vi "Protype 1.1.vi"() -> ()   [LabVIEW 2020]
uses:
  <vilib>/Utility/error.llb/DialogType.ctl
panel:
  out "MQ4 - 2":cluster{"X":dbl[], "Y":dbl[]}[](graph)
  out "MQ3 - 2":cluster{"X":dbl[], "Y":dbl[]}[](graph)
  out "Temperatur - 2":cluster{"X":dbl[], "Y":dbl[]}[](graph)
  out "Luftfeuchtigkeit - 2":cluster{"X":dbl[], "Y":dbl[]}[](graph)
  out "RAW Ethanol - 2":cluster{"X":dbl[], "Y":dbl[]}[](graph)
  out "RAW H2 - 2":cluster{"X":dbl[], "Y":dbl[]}[](graph)
  out "TVOC - 2":cluster{"X":dbl[], "Y":dbl[]}[](graph)
  out "x-y 6":dbl
  out "eCO2 - 2":cluster{"X":dbl[], "Y":dbl[]}[](graph)
  out "MH-Z19B - 2":cluster{"X":dbl[], "Y":dbl[]}[](graph)
  out "x-y 5":dbl
  out "Vernier CO2  - 2":cluster{"X":dbl[], "Y":dbl[]}[](graph) caption="XY-Graph"
  out "x-y 4":dbl
  out "Vernier Spirometer - 2":cluster{"X":dbl[], "Y":dbl[]}[](graph)
  out "x-y 3":dbl
  out "Vernier O2 - 2":cluster{"X":dbl[], "Y":dbl[]}[](graph)
  out "x-y 2":dbl
  out "Waage 2":cluster{"X":dbl[], "Y":dbl[]}[](graph) caption="XY-Graph"
  in  "Switch":bool
  in  "Graph Range":dbl=30.0
  out "x-y":dbl
  out "Luftfeuchtigkeit":dbl
  out "Temperatur":dbl
  out "Temperatur":cluster{"Y":dbl[], "Y":dbl[]}[](graph)
  out "MQ4":dbl
  out "MQ3":dbl
  out "RAW Ethanol":dbl
  out "RAW H2":dbl
  out "TVOC":dbl
  out "eCO2":dbl
  out "MHZ19b":dbl
  out "Vernier CO2":dbl
  out "Vernier Spirometer":dbl
  out "Vernier O2":dbl
  out "Waage":dbl
  in  "Filename":path=path "Komplett.xlsx" caption="Dateiname"
  in  "Record interval [ms]":u32=10000
  out "error out":errorcluster caption="Fehler (Ausgang)"
  in  "Record ?":bool=TRUE
  out "General Settings:Maximum Queue Length":u32
  out "HEMTLL - Arraygröße":i32
  out "Current Value HEMTLL":dbl[](array[numeric])
  out "Data Storage Vector - HEMTLL":dbl[][](array[numeric])
  in  "Reset MQ4":bool
  in  "Reset MQ3":bool
  in  "Reset Luftfeuchtigkeit":bool
  in  "Reset RAW Ethanol":bool
  in  "Reset RAW H2":bool
  in  "reset TVOC":bool
  in  "reset eCO2":bool
  out "Elapsed Time [s]":dbl
  out "Fehlermeldungen 8":string=" ANWEISUNGEN:\r\rAllgemeine Nutzung:  Bei der Benutzung von SubVIs, die mit den Anschlüssen \"Fehler(Eingang)\" und \"Fehler(Ausgang)\" arbeiten, platzieren Sie diesen Handler dort, wo Sie den Benutzer auf aufgetretene Fehler hinweisen möchten. In der Regel wird er am Ende eines Datenpfads als letzte Aktion des Programms aufgerufen.  Wenn der Fehlerstatus einen Fehler angibt, erzeugt der Handler eine Nachricht, die den Fehler und dessen Ursprung beschreibt.  Ist Dialogtyp = 1 (Standardeinstellung), wird die Fehlermeldung angezeigt und der Benutzer kann diese bestätigen.  Ist Dialogtyp = 2, kann der Benutzer die Meldung bestätigen oder die Programmausführung abbrechen. Der Abbruch eines Programms mit aktiver I/O wird jedoch nicht empfohlen.  Ist der Dialogtyp = 0, wird keine Meldung angezeigt; dieser Modus wird verwendet, um Fehler programmatisch zu behandeln. Aus diesem Grunde sind auch die Fehlerausgangs-Cluster mit individuellen Anschlüssen verbunden.  \r\rAndere Nutzungsmöglichkeit:\n\r\nLokales Testen.  Um einen Fehlercode eines SubVIs oder einer Funktion zu testen, die nicht mit den Fehleranschlüssen arbeitet, können der Fehlercode und ein String für \"Quelle\" mit den lokalen Eingängen \"Fehlercode\" und \"Quelle\" verbunden werden.  Wenn der Fehlerstatus keinen Fehler anzeigt und der Fehlercode ungleich 0 ist, werden der lokale Code und String \"Quelle\" ersetzt und \"Fehler?\" lautet TRUE (FEHLER)." caption="HEMTTL - Error"
  out "Gelöschte Elemente\nHEMTTL":dbl[][](array[numeric])
  out "MQ4":cluster{"Y":dbl[], "Y":dbl[]}[](graph)
  out "MQ3":cluster{"Y":dbl[], "Y":dbl[]}[](graph)
  out "Luftfeuchtigkeit":cluster{"Y":dbl[], "Y":dbl[]}[](graph)
  out "RAW Ethanol":cluster{"Y":dbl[], "Y":dbl[]}[](graph)
  out "RAW H2":cluster{"Y":dbl[], "Y":dbl[]}[](graph)
  out "TVOC":cluster{"Y":dbl[], "Y":dbl[]}[](graph)
  out "eCO2":cluster{"Y":dbl[], "Y":dbl[]}[](graph)
  in  "HEMTTL":refnum<visa-resource-name>="COM23"
  out "Vernier O2":cluster{"X":dbl[], "Y":dbl[]}[](graph) caption="XY-Graph"
  out "Gelöschte Elemente \nVernier O2":dbl[][](array[numeric])
  out "Vernier O2 - Data Storage Vector":dbl[][](array[numeric])
  out "Current Value - Vernier O2":dbl[](array[numeric])
  out "Vernier O2":i32
  in  "Reset Vernier O2":bool caption="Zurücksetzen"
  out "Fehlermeldungen 7":string=" ANWEISUNGEN:\r\rAllgemeine Nutzung:  Bei der Benutzung von SubVIs, die mit den Anschlüssen \"Fehler(Eingang)\" und \"Fehler(Ausgang)\" arbeiten, platzieren Sie diesen Handler dort, wo Sie den Benutzer auf aufgetretene Fehler hinweisen möchten. In der Regel wird er am Ende eines Datenpfads als letzte Aktion des Programms aufgerufen.  Wenn der Fehlerstatus einen Fehler angibt, erzeugt der Handler eine Nachricht, die den Fehler und dessen Ursprung beschreibt.  Ist Dialogtyp = 1 (Standardeinstellung), wird die Fehlermeldung angezeigt und der Benutzer kann diese bestätigen.  Ist Dialogtyp = 2, kann der Benutzer die Meldung bestätigen oder die Programmausführung abbrechen. Der Abbruch eines Programms mit aktiver I/O wird jedoch nicht empfohlen.  Ist der Dialogtyp = 0, wird keine Meldung angezeigt; dieser Modus wird verwendet, um Fehler programmatisch zu behandeln. Aus diesem Grunde sind auch die Fehlerausgangs-Cluster mit individuellen Anschlüssen verbunden.  \r\rAndere Nutzungsmöglichkeit:\n\r\nLokales Testen.  Um einen Fehlercode eines SubVIs oder einer Funktion zu testen, die nicht mit den Fehleranschlüssen arbeitet, können der Fehlercode und ein String für \"Quelle\" mit den lokalen Eingängen \"Fehlercode\" und \"Quelle\" verbunden werden.  Wenn der Fehlerstatus keinen Fehler anzeigt und der Fehlercode ungleich 0 ist, werden der lokale Code und String \"Quelle\" ersetzt und \"Fehler?\" lautet TRUE (FEHLER)."
  out "Vernier Spirometer":cluster{"X":dbl[], "Y":dbl[]}[](graph) caption="XY-Graph"
  out "Gelöschte Elemente \nVernier Spirometer":dbl[][](array[numeric])
  out "Data Storage vector - \nVernier Spirometer":dbl[][](array[numeric])
  out "Current Value - \nVernier Spirometer":dbl[](array[numeric])
  out "Vernier Spirometer-\n Array Größe":i32
  in  "Reset Spirometer":bool caption="Zurücksetzen"
  out "Fehlermeldungen 6":string=" ANWEISUNGEN:\r\rAllgemeine Nutzung:  Bei der Benutzung von SubVIs, die mit den Anschlüssen \"Fehler(Eingang)\" und \"Fehler(Ausgang)\" arbeiten, platzieren Sie diesen Handler dort, wo Sie den Benutzer auf aufgetretene Fehler hinweisen möchten. In der Regel wird er am Ende eines Datenpfads als letzte Aktion des Programms aufgerufen.  Wenn der Fehlerstatus einen Fehler angibt, erzeugt der Handler eine Nachricht, die den Fehler und dessen Ursprung beschreibt.  Ist Dialogtyp = 1 (Standardeinstellung), wird die Fehlermeldung angezeigt und der Benutzer kann diese bestätigen.  Ist Dialogtyp = 2, kann der Benutzer die Meldung bestätigen oder die Programmausführung abbrechen. Der Abbruch eines Programms mit aktiver I/O wird jedoch nicht empfohlen.  Ist der Dialogtyp = 0, wird keine Meldung angezeigt; dieser Modus wird verwendet, um Fehler programmatisch zu behandeln. Aus diesem Grunde sind auch die Fehlerausgangs-Cluster mit individuellen Anschlüssen verbunden.  \r\rAndere Nutzungsmöglichkeit:\n\r\nLokales Testen.  Um einen Fehlercode eines SubVIs oder einer Funktion zu testen, die nicht mit den Fehleranschlüssen arbeitet, können der Fehlercode und ein String für \"Quelle\" mit den lokalen Eingängen \"Fehlercode\" und \"Quelle\" verbunden werden.  Wenn der Fehlerstatus keinen Fehler anzeigt und der Fehlercode ungleich 0 ist, werden der lokale Code und String \"Quelle\" ersetzt und \"Fehler?\" lautet TRUE (FEHLER)."
  out "MH-Z19B":cluster{"X":dbl[], "Y":dbl[]}[](graph) caption="XY-Graph"
  out "Gelöschte Elemente \nMHZ19b":dbl[][](array[numeric])
  out "MHZ19b":dbl[][](array[numeric])
  out "Current Value - MHZ19b":dbl[](array[numeric])
  out "MHZ19b - Arraygröße":i32
  in  "Reset MHZ19b":bool caption="Zurücksetzen"
  out "Fehlermeldungen 5":string=" ANWEISUNGEN:\r\rAllgemeine Nutzung:  Bei der Benutzung von SubVIs, die mit den Anschlüssen \"Fehler(Eingang)\" und \"Fehler(Ausgang)\" arbeiten, platzieren Sie diesen Handler dort, wo Sie den Benutzer auf aufgetretene Fehler hinweisen möchten. In der Regel wird er am Ende eines Datenpfads als letzte Aktion des Programms aufgerufen.  Wenn der Fehlerstatus einen Fehler angibt, erzeugt der Handler eine Nachricht, die den Fehler und dessen Ursprung beschreibt.  Ist Dialogtyp = 1 (Standardeinstellung), wird die Fehlermeldung angezeigt und der Benutzer kann diese bestätigen.  Ist Dialogtyp = 2, kann der Benutzer die Meldung bestätigen oder die Programmausführung abbrechen. Der Abbruch eines Programms mit aktiver I/O wird jedoch nicht empfohlen.  Ist der Dialogtyp = 0, wird keine Meldung angezeigt; dieser Modus wird verwendet, um Fehler programmatisch zu behandeln. Aus diesem Grunde sind auch die Fehlerausgangs-Cluster mit individuellen Anschlüssen verbunden.  \r\rAndere Nutzungsmöglichkeit:\n\r\nLokales Testen.  Um einen Fehlercode eines SubVIs oder einer Funktion zu testen, die nicht mit den Fehleranschlüssen arbeitet, können der Fehlercode und ein String für \"Quelle\" mit den lokalen Eingängen \"Fehlercode\" und \"Quelle\" verbunden werden.  Wenn der Fehlerstatus keinen Fehler anzeigt und der Fehlercode ungleich 0 ist, werden der lokale Code und String \"Quelle\" ersetzt und \"Fehler?\" lautet TRUE (FEHLER)."
  in  "Reset all":bool caption="Zurücksetzen"
  out "Waage":cluster{"X":dbl[], "Y":dbl[]}[](graph)=[{"X"=array[301 elements], "Y"=[7.03, 7.14, 7.27, 7.31, 7.28, 7.21, 7.21, 7.24, 7.21, 7.21, 7.21, 7.25, 7.25, 7.15, 7.16, 7.3, 7.41, 7.35, 7.38, 7.36, 7.35, 7.43, 7.46, 7.43, 7.48, 7.54, 7.6, 7.52, 7.4, 7.38, 7.37, 7.4, 7.47, 7.51, 7.51, 7.42, 7.45, 7.48, 7.42, 7.39, 7.49, 7.57, 7.51, 7.55, 7.56, 7.54, 7.55, 7.45, 7.42, 7.46, 7.43, 7.46, 7.55, 7.59, 7.56, 7.58, 7.64, 7.61, 7.55, 7.47, 7.42, 7.46, 7.58, 7.6, 7.51, 7.42, 7.39, 7.42, 7.5, 7.54, 7.52, 7.58, 7.73, 7.73, 7.53, 7.5, 7.52, 7.5, 7.52, 7.49, 7.51, 7.59, 7.57, 7.47, 7.46, 7.53, 7.51, 7.56, 7.5, 7.45, 7.61, 7.65, 7.59, 7.54, 7.57, 7.63, 7.69, 7.67, 7.59, 7.61, 7.56, 7.46, 7.47, 7.48, 7.51, 7.63, 7.58, 7.5, 7.66, 7.71, 7.72, 7.67, 7.58, 7.71, 7.65, 7.64, 7.71, 7.64, 7.59, 7.58, 7.56, 7.53, 7.54, 7.68, 7.79, 7.69, 7.61, 7.67, 7.68, 7.68, 7.62, 7.67, 7.8, 7.76, 7.72, 7.73, 7.75, 7.73, 7.73, 7.78, 7.78, 7.72, 7.78, 7.81, 7.76, 7.86, 7.86, 7.81, 7.81, 7.85, 7.85, 7.8, 7.85, 7.88, 7.85, 7.83, 7.77, 7.72, 7.8, 7.83, 7.71, 7.65, 7.68, 7.68, 7.66, 7.67, 7.74, 7.74, 7.82, 7.8, 7.7, 7.68, 7.74, 7.84, 7.87, 7.89, 7.89, 7.79, 7.73, 7.65, 7.72, 7.91, 7.96, 8.03, 8.0, 7.92, 7.91, 7.95, 7.97, 8.04, 8.08, 8.07, 8.09, 7.99, 7.99, 8.04, 8.0, 7.95, 7.99, 7.94, 7.89, 8.02, 7.98, 8.07, 8.18, 8.15, 8.12, 8.0, 7.91, 8.06, 8.19, 8.19, 8.16, 8.07, 8.03, 7.99, 7.91, 7.98, 8.03, 8.02, 7.98, 7.87, 7.75, 7.76, 7.96, 8.01, 8.04, 7.95, 7.9, 8.01, 8.02, 7.99, 8.11, 8.13, 8.0, 8.09, 8.16, 8.05, 8.12, 8.19, 8.14, 8.25, 8.2, 8.02, 8.04, 8.12, 8.12, 8.12, 8.08, 8.1, 7.96, 7.97, 8.02, 8.04, 8.06, 8.12, 8.19, 8.27, 8.28, 8.18, 8.14, 8.09, 8.1, 8.19, 8.24, 8.19, 8.15, 8.14, 8.21, 8.23, 8.15, 8.09, 8.01, 7.95, 8.03, 8.1, 8.16, 8.23, 8.34, 8.38, 8.33, 8.22, 8.19, 8.23, 8.21, 8.26, 8.29, 8.3, 8.19, 8.2, 8.28, 8.31, 8.35, 8.31, 8.33, 8.27, 8.17, 8.23, 8.25, 8.29, 8.24]}] caption="XY-Graph"
  out "Gelöschte Elemente \nWaage":dbl[][](array[numeric])
  out "Waage - Data Storage Vector":dbl[][](array[numeric])
  out "Waage - Current Value":dbl[](array[numeric])
  out "Waage":i32
  in  "Arraygröße":i32=10
  in  "Reset Waage":bool caption="Zurücksetzen"
  in  "Reset Vernier CO2":bool caption="Zurücksetzen"
  in  "Byte-Anzahl":u32=10000
  out "Vernier CO2":cluster{"X":dbl[], "Y":dbl[]}[](graph) caption="XY-Graph"
  out "Gelöschte Elemente \nVernier CO2":dbl[][](array[numeric])
  out "Data Storage Vector - Vernier CO2":dbl[][](array[numeric])
  out "Current Value Vernier CO2":dbl[](array[numeric])
  out "Vernier CO2":i32
  out "Fehlermeldungen 4":string=" ANWEISUNGEN:\r\rAllgemeine Nutzung:  Bei der Benutzung von SubVIs, die mit den Anschlüssen \"Fehler(Eingang)\" und \"Fehler(Ausgang)\" arbeiten, platzieren Sie diesen Handler dort, wo Sie den Benutzer auf aufgetretene Fehler hinweisen möchten. In der Regel wird er am Ende eines Datenpfads als letzte Aktion des Programms aufgerufen.  Wenn der Fehlerstatus einen Fehler angibt, erzeugt der Handler eine Nachricht, die den Fehler und dessen Ursprung beschreibt.  Ist Dialogtyp = 1 (Standardeinstellung), wird die Fehlermeldung angezeigt und der Benutzer kann diese bestätigen.  Ist Dialogtyp = 2, kann der Benutzer die Meldung bestätigen oder die Programmausführung abbrechen. Der Abbruch eines Programms mit aktiver I/O wird jedoch nicht empfohlen.  Ist der Dialogtyp = 0, wird keine Meldung angezeigt; dieser Modus wird verwendet, um Fehler programmatisch zu behandeln. Aus diesem Grunde sind auch die Fehlerausgangs-Cluster mit individuellen Anschlüssen verbunden.  \r\rAndere Nutzungsmöglichkeit:\n\r\nLokales Testen.  Um einen Fehlercode eines SubVIs oder einer Funktion zu testen, die nicht mit den Fehleranschlüssen arbeitet, können der Fehlercode und ein String für \"Quelle\" mit den lokalen Eingängen \"Fehlercode\" und \"Quelle\" verbunden werden.  Wenn der Fehlerstatus keinen Fehler anzeigt und der Fehlercode ungleich 0 ist, werden der lokale Code und String \"Quelle\" ersetzt und \"Fehler?\" lautet TRUE (FEHLER)."
  in  "MHZ19b":refnum<visa-resource-name>="COM11"
  in  "Vernier Co2":refnum<visa-resource-name>="COM6"
  in  "Vernier Spirometer":refnum<visa-resource-name>="COM4"
  in  "Vernier O2":refnum<visa-resource-name>="COM7"
  out "Start":timestamp
  in  "Tara":bool
  in  "Kalibrierung [2000 g]":bool
  out "Fehlermeldungen":string=" ANWEISUNGEN:\r\rAllgemeine Nutzung:  Bei der Benutzung von SubVIs, die mit den Anschlüssen \"Fehler(Eingang)\" und \"Fehler(Ausgang)\" arbeiten, platzieren Sie diesen Handler dort, wo Sie den Benutzer auf aufgetretene Fehler hinweisen möchten. In der Regel wird er am Ende eines Datenpfads als letzte Aktion des Programms aufgerufen.  Wenn der Fehlerstatus einen Fehler angibt, erzeugt der Handler eine Nachricht, die den Fehler und dessen Ursprung beschreibt.  Ist Dialogtyp = 1 (Standardeinstellung), wird die Fehlermeldung angezeigt und der Benutzer kann diese bestätigen.  Ist Dialogtyp = 2, kann der Benutzer die Meldung bestätigen oder die Programmausführung abbrechen. Der Abbruch eines Programms mit aktiver I/O wird jedoch nicht empfohlen.  Ist der Dialogtyp = 0, wird keine Meldung angezeigt; dieser Modus wird verwendet, um Fehler programmatisch zu behandeln. Aus diesem Grunde sind auch die Fehlerausgangs-Cluster mit individuellen Anschlüssen verbunden.  \r\rAndere Nutzungsmöglichkeit:\n\r\nLokales Testen.  Um einen Fehlercode eines SubVIs oder einer Funktion zu testen, die nicht mit den Fehleranschlüssen arbeitet, können der Fehlercode und ein String für \"Quelle\" mit den lokalen Eingängen \"Fehlercode\" und \"Quelle\" verbunden werden.  Wenn der Fehlerstatus keinen Fehler anzeigt und der Fehlercode ungleich 0 ist, werden der lokale Code und String \"Quelle\" ersetzt und \"Fehler?\" lautet TRUE (FEHLER)."
  in  "Waage":refnum<visa-resource-name>="COM9"
  # "General settings"
  # "Vernier O2"
  # "Waage"
  # "Current Value       |   Data storage vector       |    Deleted elements         |    Error                                                              | Arraysize"
  # "Current Value       |   Data storage vector       |    Deleted elements         |    Error                                                              | Arraysize"
  # "COM Settings"
  # "Vernier Spirometer"
  # "Vernier CO2"
  # "Current Value       |   Data storage vector       |    Deleted elements         |    Error                                                              | Arraysize"
  # "Current Value       |   Data storage vector       |    Deleted elements         |    Error                                                              | Arraysize"
  # "MHZ19b - CO2"
  # "Current Value       |   Data storage vector       |    Deleted elements         |    Error                                                              | Arraysize"
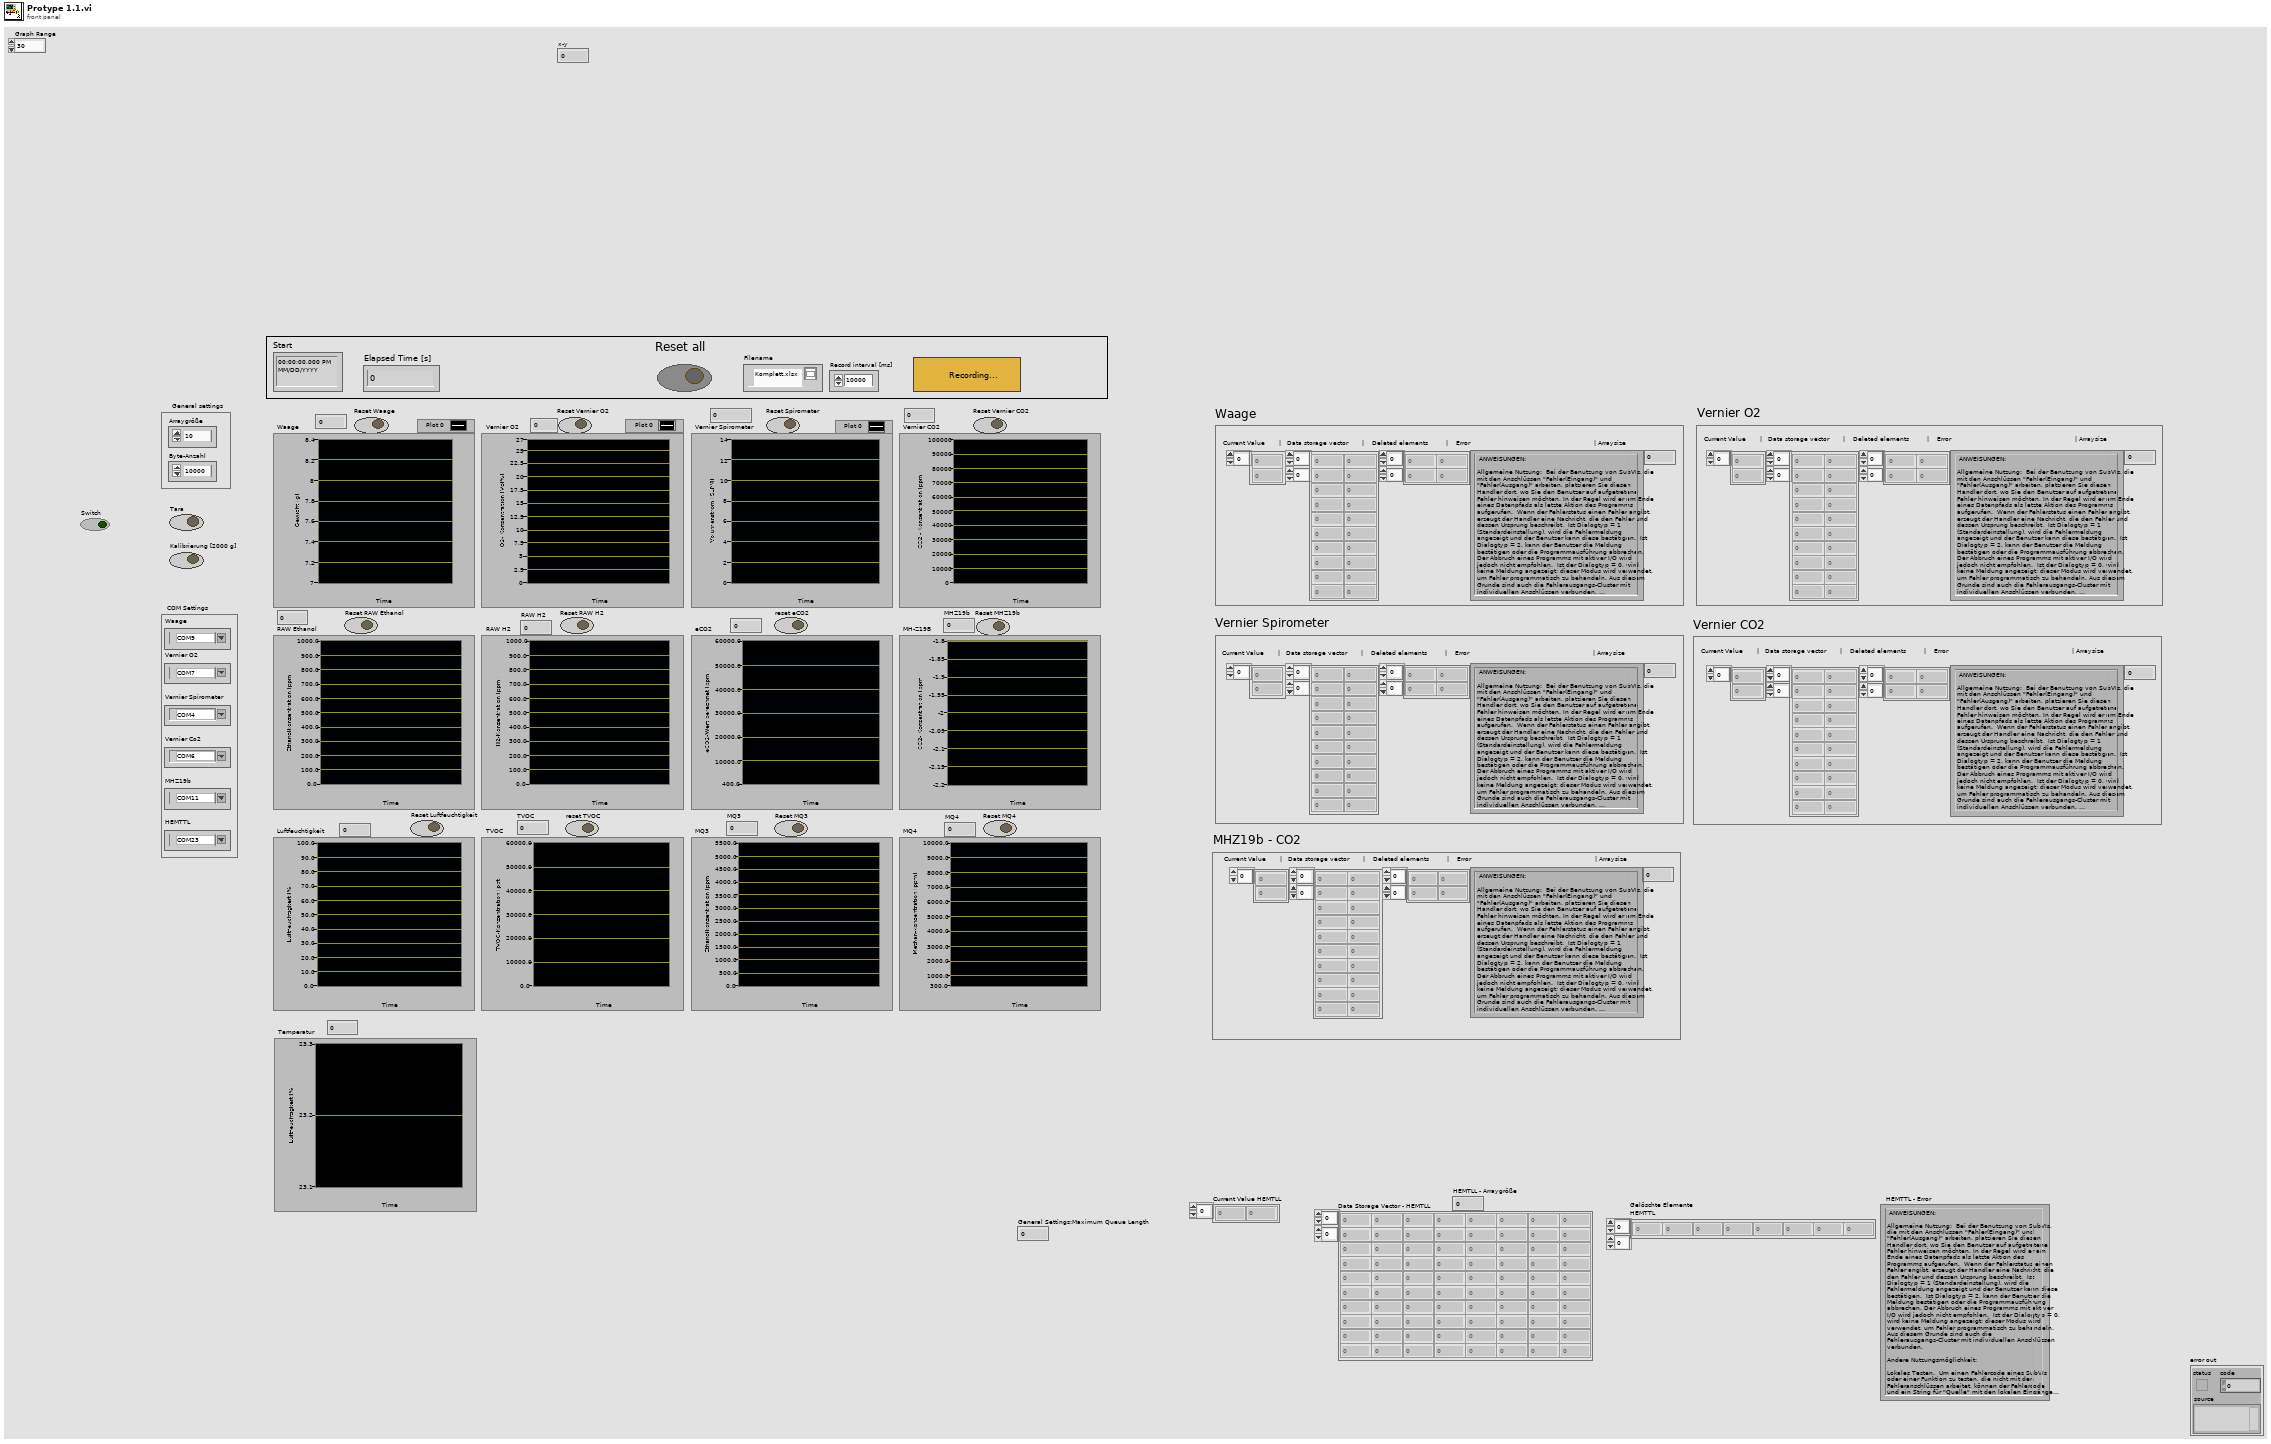
[diagram p1: front panel]
types:
  T1 = typedef "DialogType.ctl" = u16
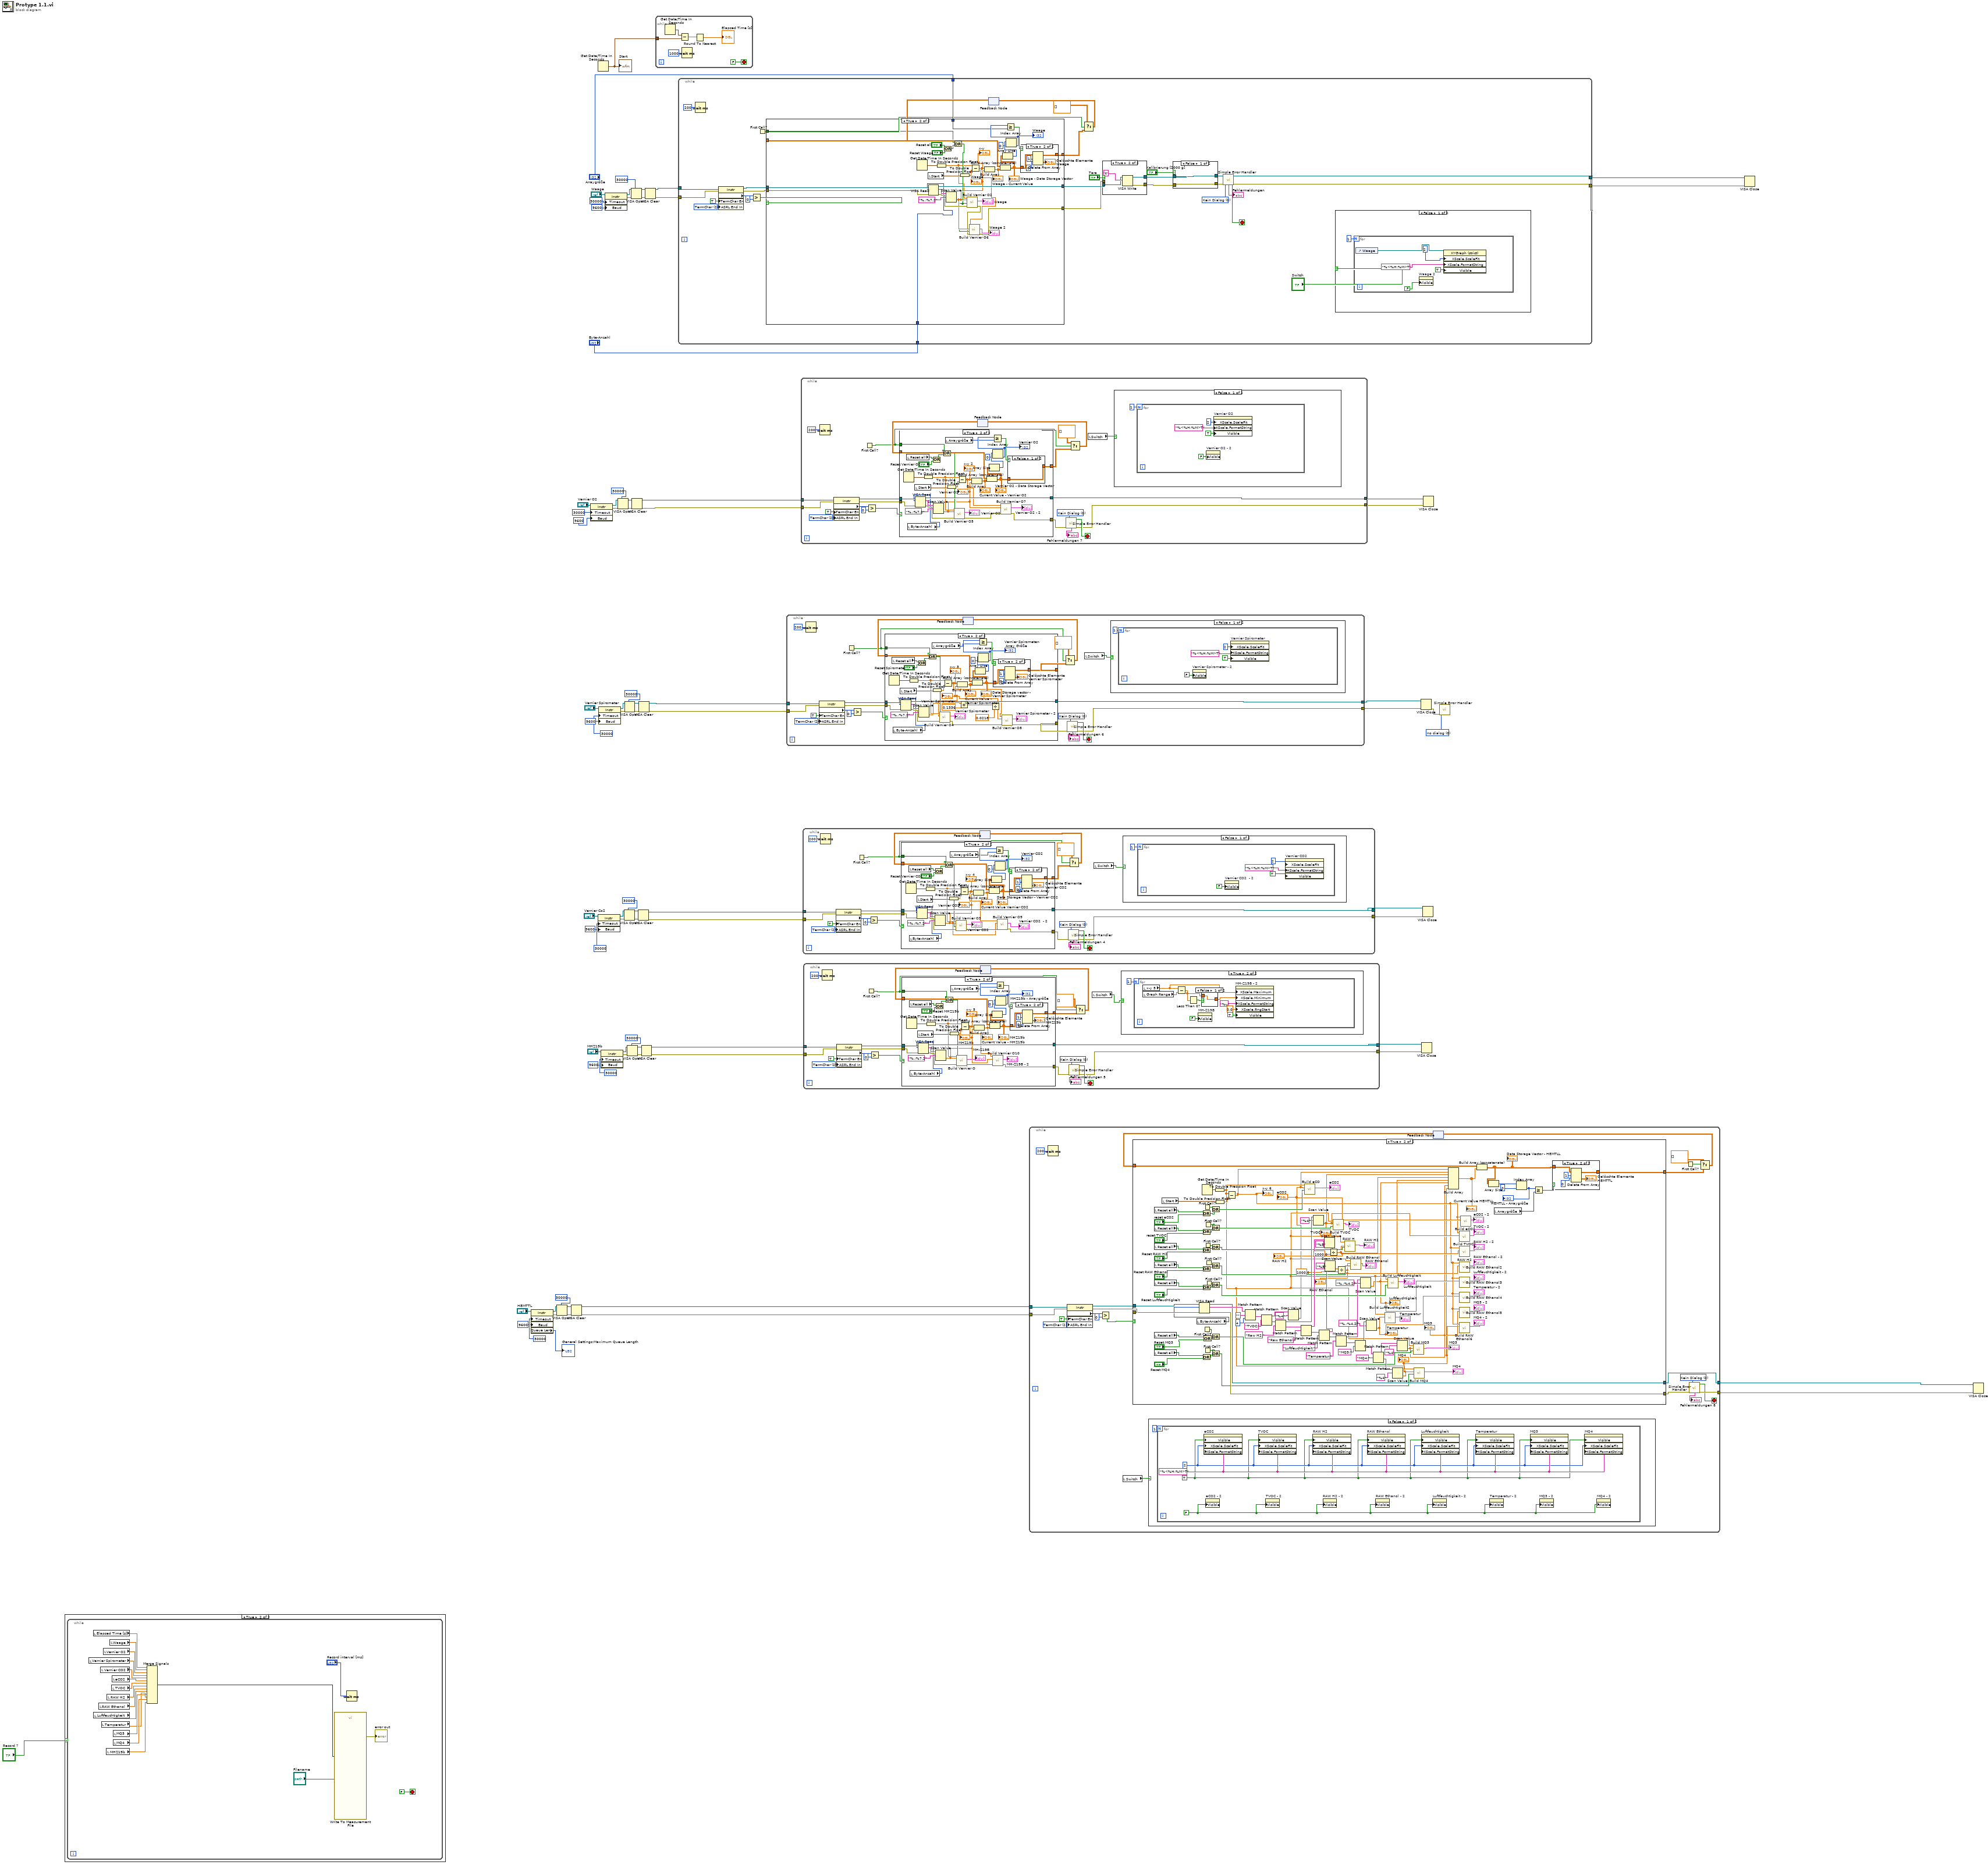
[diagram p0: block diagram]
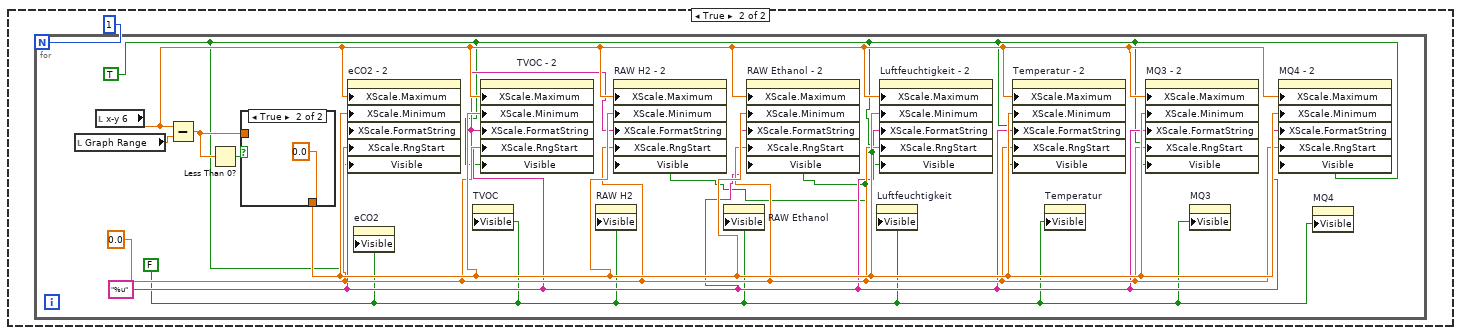
[diagram p3: hidden frame]
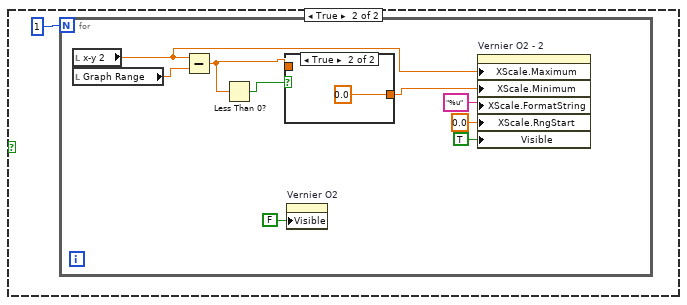
[diagram p7: hidden frame]
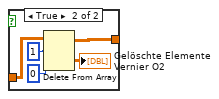
[diagram p10: hidden frame]
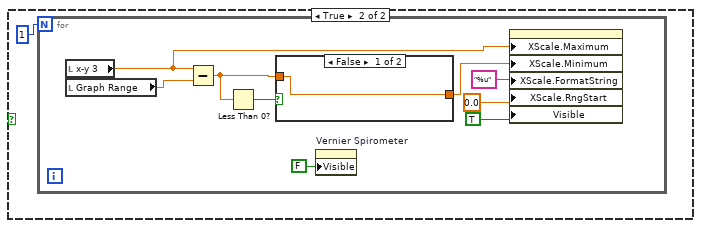
[diagram p11: hidden frame]
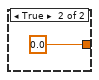
[diagram p12: hidden frame]
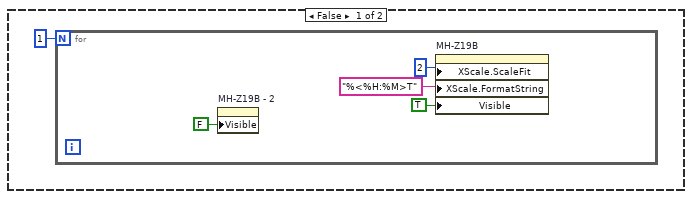
[diagram p15: hidden frame]
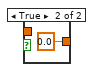
[diagram p16: hidden frame]
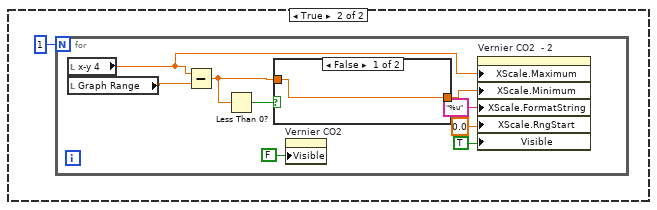
[diagram p19: hidden frame]
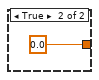
[diagram p20: hidden frame]
diagram:
  w1 = T1 0 items=["no dialog", "OK message", "continue or stop message", "OK message + warnings", "continue/stop + warnings"] ("type of dialog (OK msg:1)")
  n1 = case shown="True" "Record ?" {
    frame False {
    }
    frame True {
      n2 = while {
        stop <- FALSE stop-if-true
        n3 = local read "Vernier Spirometer"() -> (w91:dbl)
        n4 = local read "Elapsed Time [s]"() -> (w94:dbl)
        n5 = local read "Luftfeuchtigkeit"() -> (w80:dbl)
        n6 = local read "RAW Ethanol"() -> (w86:dbl)
        n7 = local read "Vernier CO2"() -> (w90:dbl)
        n8 = local read "Temperatur"() -> (w81:dbl)
        n9 = local read "Vernier O2"() -> (w92:dbl)
        n10 = local read "MHZ19b"() -> (w82:dbl)
        n11 = local read "RAW H2"() -> (w87:dbl)
        n12 = local read "Waage"() -> (w93:dbl)
        n13 = local read "TVOC"() -> (w88:dbl)
        n14 = local read "eCO2"() -> (w89:dbl)
        n15 = local read "MQ3"() -> (w84:dbl)
        n16 = local read "MQ4"() -> (w83:dbl)
        n17 = Merge Signals(w94, w93, w92, w91, w90, w89, w88, w87, w86, w80, w81, w84, w83, w82) -> (w85:dynamicdata)
        n18 = call "Write To Measurement File"("Signals"=w85, "Filename"="Filename") -> ("error out"=→"error out":errorcluster)  [unwired: 15 in, 2 out]
        n19 = Wait (ms)(milliseconds to wait="Record interval [ms]") -> ()  [unwired: 1 out]
      }
    }
  }
  n20 = property class="Instr"(reference="HEMTTL", "Timeout"=u32 30000 ("General Settings:Timeout Value"), "Baud"=u32 9600 ("Serial Settings:Baud Rate")) -> (reference out=w16:refnum<visa-resource-name>, error out=w17:errorcluster, "Queue Len"=→"General Settings:Maximum Queue Length":u32)  [unwired: 1 in]
  n21 = VISA Open(timeout (0)=u32 30000 ("VISA: Timeout bei Öffnen (0)"), error in (no error)=w17, VISA resource name=w16) -> (VISA resource name=w13:refnum<visa-resource-name>, error out=w14:errorcluster)  [unwired: 2 in]
  n22 = VISA Clear(VISA resource name=w13, error in (no error)=w14) -> (VISA resource name out=w4:refnum<visa-resource-name>, error out=w3:errorcluster)
  n23 = property class="Instr"(reference="Vernier O2", "Timeout"=u32 30000 ("General Settings:Timeout Value"), "Baud"=u32 9600 ("Serial Settings:Baud Rate")) -> (reference out=w68:refnum<visa-resource-name>, error out=w69:errorcluster)  [unwired: 1 in]
  n24 = Get Date/Time In Seconds() -> (seconds since 1Jan1904=w7:timestamp)
  "Start" <- w7
  n25 = property class="Instr"(reference="Vernier Co2", "Timeout"=u32 30000 ("General Settings:Timeout Value"), "Baud"=u32 9600 ("Serial Settings:Baud Rate")) -> (reference out=w56:refnum<visa-resource-name>, error out=w57:errorcluster)  [unwired: 1 in]
  n26 = property class="Instr"(reference="Vernier Spirometer", "Timeout"=u32 30000 ("General Settings:Timeout Value"), "Baud"=u32 9600 ("Serial Settings:Baud Rate")) -> (reference out=w62:refnum<visa-resource-name>, error out=w63:errorcluster)  [unwired: 1 in]
  n27 = property class="Instr"(reference="MHZ19b", "Timeout"=u32 30000 ("General Settings:Timeout Value"), "Baud"=u32 9600 ("Serial Settings:Baud Rate")) -> (reference out=w50:refnum<visa-resource-name>, error out=w51:errorcluster)  [unwired: 1 in]
  n28 = property class="Instr"(reference="Waage", "Timeout"=u32 30000 ("General Settings:Timeout Value"), "Baud"=u32 9600 ("Serial Settings:Baud Rate")) -> (reference out=w76:refnum<visa-resource-name>, error out=w77:errorcluster)  [unwired: 1 in]
  n29 = VISA Open(timeout (0)=u32 30000 ("VISA: Timeout bei Öffnen (0)"), error in (no error)=w69, VISA resource name=w68) -> (VISA resource name=w65:refnum<visa-resource-name>, error out=w66:errorcluster)  [unwired: 2 in]
  n30 = VISA Open(timeout (0)=u32 30000 ("VISA: Timeout bei Öffnen (0)"), error in (no error)=w57, VISA resource name=w56) -> (VISA resource name=w53:refnum<visa-resource-name>, error out=w54:errorcluster)  [unwired: 2 in]
  n31 = VISA Open(timeout (0)=u32 30000 ("VISA: Timeout bei Öffnen (0)"), error in (no error)=w63, VISA resource name=w62) -> (VISA resource name=w59:refnum<visa-resource-name>, error out=w60:errorcluster)  [unwired: 2 in]
  n32 = VISA Open(timeout (0)=u32 30000 ("VISA: Timeout bei Öffnen (0)"), error in (no error)=w51, VISA resource name=w50) -> (VISA resource name=w47:refnum<visa-resource-name>, error out=w48:errorcluster)  [unwired: 2 in]
  n33 = VISA Open(timeout (0)=u32 30000 ("VISA: Timeout bei Öffnen (0)"), error in (no error)=w77, VISA resource name=w76) -> (VISA resource name=w73:refnum<visa-resource-name>, error out=w74:errorcluster)  [unwired: 2 in]
  n34 = VISA Clear(VISA resource name=w65, error in (no error)=w66) -> (VISA resource name out=w28:refnum<visa-resource-name>, error out=w27:errorcluster)
  n35 = VISA Clear(VISA resource name=w53, error in (no error)=w54) -> (VISA resource name out=w42:refnum<visa-resource-name>, error out=w41:errorcluster)
  n36 = VISA Clear(VISA resource name=w59, error in (no error)=w60) -> (VISA resource name out=w30:refnum<visa-resource-name>, error out=w29:errorcluster)
  n37 = VISA Clear(VISA resource name=w47, error in (no error)=w48) -> (VISA resource name out=w36:refnum<visa-resource-name>, error out=w35:errorcluster)
  n38 = VISA Clear(VISA resource name=w73, error in (no error)=w74) -> (VISA resource name out=w71:refnum<visa-resource-name>, error out=w70:errorcluster)
  n39 = while {
    tunnel: w7 -> [w102]
    stop <- FALSE stop-if-true
    n40 = Get Date/Time In Seconds() -> (seconds since 1Jan1904=w103:timestamp)
    n41 = Subtract(x=w103, y=w102) -> (x-y=w100:dbl)
    n42 = Wait (ms)(milliseconds to wait=u32 1000 ("Zu wartende ms")) -> ()  [unwired: 1 out]
    n43 = Round To Nearest(number=w100) -> (nearest integer value=→"Elapsed Time [s]":dbl)
  }
  n44 = while {
    tunnel: w71 -> [w120]
    tunnel: w70 -> [w119]
    tunnel: [w129] -> w79
    tunnel: [w127] -> w78
    tunnel: "Byte-Anzahl" -> [w112]
    tunnel: "Arraygröße" -> [w111]
    stop <- w133 stop-if-true
    w123 = u16 2 items=["None", "Last Bit", "TermChar"] ("Serial Settings:End Mode for Reads")
    w126 = T1 0 items=["Kein Dialog", "OK-Meldung", "Dialog zum Fortsetzen oder Anhalten", "OK-Meldung + Warnungen", "Weiter/Stopp + Warnung"] ("type of dialog (OK msg:1)")
    n45 = Wait (ms)(milliseconds to wait=u32 200) -> ()  [unwired: 1 out]
    n46 = property class="Instr"(reference=w120, error in=w119, "TermChar En"=TRUE ("Message Based Settings:Termination Character Enable"), "ASRL End In"=w123) -> (reference out=w116:refnum<visa-resource-name>, error out=w115:errorcluster, "Serial Settings:Number of Bytes at Serial Port"=w122:u32)
    n47 = Greater?(x=w122, y=u32 0) -> (0:w110:bool)
    n48 = First Call?() -> (First Call?: T/F=w106:bool)
    n49 = feedback #1() -> (w117:dbl[][])  [unwired: 1 in]
    n50 = case shown="True" w110 {
      tunnel: w116 -> [w156 w187]
      tunnel: w115 -> [w155 w186]
      tunnel: [w156 w185] -> w113
      tunnel: [w155 w159] -> w114
      tunnel: [w154 w171] -> w109
      tunnel: w117 -> [w154 w170]
      tunnel: w112 -> [_ w166]
      tunnel: w111 -> [_ w165]
      tunnel: w106 -> [_ w164]
      frame False {
      }
      frame True {
        n51 = Get Date/Time In Seconds() -> (seconds since 1Jan1904=w182:timestamp)
        n52 = local read "Start"() -> (w181:timestamp)
        n53 = VISA Read(VISA resource name=w187, byte count=w166, error in (no error)=w186) -> (VISA resource name out=w185:refnum<visa-resource-name>, read buffer=w184:string, error out=w178:errorcluster)  [unwired: 1 out]
        n54 = To Double Precision Float(number=w182) -> (double precision float=w158:dbl)
        n55 = Or(x="Reset all", y="Reset Waage") -> (x .or. y?=w167:bool)
        n56 = Scan Value(string=w184, format string="%.;%7.2" ("Format-String")) -> (value=w162:dbl)  [unwired: 1 in, 1 out]
        "Waage" <- w162
        n57 = Or(x=w164, y=w167) -> (x .or. y?=w161:bool)
        n58 = To Double Precision Float(number=w181) -> (double precision float=w179:dbl)
        n59 = call "Build Vernier O2"("error in (no error)"=w178, "Reset"=w161, "Y Input"=w162, "X Input"=w158) -> ("error out"=w160:errorcluster, "XY Graph"=→"Waage":cluster{"X":dbl[], "Y":dbl[]}[])  [unwired: 6 in]
        n60 = Subtract(x=w158, y=w179) -> (x-y=w157:dbl)
        "x-y" <- w157
        n61 = call "Build Vernier O6"("error in (no error)"=w160, "Reset"=w161, "Y Input"=w162, "X Input"=w157) -> ("error out"=w159:errorcluster, "XY Graph"=→"Waage 2":cluster{"X":dbl[], "Y":dbl[]}[])  [unwired: 6 in]
        n62 = Build Array(w157, w162) -> (w177:dbl[])
        "Waage - Current Value" <- w177
        n63 = Build Array (concatenate)(w170, w177) -> (w176:dbl[][])
        "Waage - Data Storage Vector" <- w176
        n64 = Array Size(array=w176) -> (size(s)=w175:i32[])
        n65 = Index Array(array=w175, index=0 ("Index")) -> (element=w173:i32)
        "Waage" <- w173
        n66 = Greater Or Equal?(x=w173, y=w165) -> (x >= y?=w172:bool)
        n67 = case shown="True" w172 {
          tunnel: w176 -> [w188 w193]
          tunnel: [w188 w192] -> w171
          frame False {
          }
          frame True {
            n68 = Delete From Array(array=w193, length=1 ("Länge"), index (row)=0 ("Index")) -> (deleted portion=→"Gelöschte Elemente \nWaage":dbl[][], array with subset deleted=w192:dbl[][])  [unwired: 1 in]
          }
        }
      }
    }
    n69 = Select(t=dbl[][] [], s=w106, f=w109) -> (s? t:f=w108:dbl[][])
    n70 = feedback-in #1(w108) -> ()
    n71 = case shown="True" "Tara" {
      tunnel: w113 -> [w201 w205]
      tunnel: w114 -> [w202 _]
      tunnel: [w201 w204] -> w130
      tunnel: [w202 w203] -> w118
      frame False {
      }
      frame True {
        n72 = VISA Write(VISA resource name=w205, write buffer="t" ("Schreibpuffer")) -> (VISA resource name out=w204:refnum<visa-resource-name>, error out=w203:errorcluster)  [unwired: 1 in, 1 out]
      }
    }
    n73 = case shown="False" "Kalibrierung [2000 g]" {
      tunnel: w130 -> [w194 w199]
      tunnel: w118 -> [w195 w198]
      tunnel: [w194 w197] -> w129
      tunnel: [w195 w196] -> w128
      frame False {
      }
      frame True {
        n74 = VISA Write(VISA resource name=w199, write buffer="r" ("Schreibpuffer"), error in (no error)=w198) -> (VISA resource name out=w197:refnum<visa-resource-name>, error out=w196:errorcluster)  [unwired: 1 out]
      }
    }
    n75 = call <vilib>:"Simple Error Handler.vi"("type of dialog (OK msg:1)"=w126, "error in (no error)"=w128) -> ("error?"=w133:bool, "error out"=w127:errorcluster, "message"=→"Fehlermeldungen":string)  [unwired: 5 out]
    n76 = case shown="False" "Switch" {
      frame False {
        n77 = for {
          N: 1 -> [_]
          n78 = control-ref of="Waage"() -> (w137:refnum<vi>)
          n79 = property on="Waage 2" class="XYGraph (strict)"("Visible"=FALSE) -> ()  [unwired: 2 in, 2 out]
          n80 = property on="Property Node" class="XYGraph (strict)"(reference=w137, "XScale.ScaleFit"=u8 2 ("X Scale.Scale Fit"), "XScale.FormatString"="%<%H:%M>T" ("X Scale.Format String"), "Visible"=TRUE) -> ()  [unwired: 1 in, 2 out]
        }
      }
      frame True {
        n81 = for {
          N: 1 -> [_]
          n82 = local read "x-y"() -> (w142:dbl)
          n83 = Subtract(x=w142, y="Graph Range") -> (x-y=w149:dbl)
          n84 = Less Than 0?(x=w149) -> (x < 0?=w150:bool)
          n85 = control-ref of="Waage 2"() -> (w144:refnum<vi>)
          n86 = case shown="False" w150 {
            tunnel: w149 -> [w152 _]
            tunnel: [w152 0.0] -> w148
            frame False {
            }
            frame True {
            }
          }
          n87 = property on="Waage" class="XYGraph (strict)"("Visible"=FALSE) -> ()  [unwired: 2 in, 2 out]
          n88 = property on="Property Node" class="XYGraph (strict)"(reference=w144, "XScale.Maximum"=w142, "XScale.Minimum"=w148, "XScale.RngStart"=0.0 ("Y Scale.Range:Minimum"), "XScale.FormatString"="%u" ("X Scale.Format String"), "Visible"=TRUE) -> ()  [unwired: 1 in, 2 out]
        }
      }
    }
  }
  n89 = while {
    tunnel: w30 -> [w227]
    tunnel: w29 -> [w226]
    tunnel: [w220] -> w32
    tunnel: [w215] -> w31
    stop <- w217 stop-if-true
    w216 = T1 0 items=["Kein Dialog", "OK-Meldung", "Dialog zum Fortsetzen oder Anhalten", "OK-Meldung + Warnungen", "Weiter/Stopp + Warnung"] ("type of dialog (OK msg:1)")
    w225 = u16 2 items=["None", "Last Bit", "TermChar"] ("Serial Settings:End Mode for Reads")
    n90 = Wait (ms)(milliseconds to wait=u32 200) -> ()  [unwired: 1 out]
    n91 = property class="Instr"(reference=w227, error in=w226, "TermChar En"=TRUE ("Message Based Settings:Termination Character Enable"), "ASRL End In"=w225) -> (reference out=w222:refnum<visa-resource-name>, error out=w221:errorcluster, "Serial Settings:Number of Bytes at Serial Port"=w224:u32)
    n92 = First Call?() -> (First Call?: T/F=w209:bool)
    n93 = Greater?(x=w224, y=u32 0) -> (0:w212:bool)
    n94 = feedback #2() -> (w214:dbl[][])  [unwired: 1 in]
    n95 = case shown="True" w212 {
      tunnel: w222 -> [w248 w283]
      tunnel: w221 -> [w247 w282]
      tunnel: [w248 w281] -> w220
      tunnel: [w247 w249] -> w219
      tunnel: [w246 w266] -> w211
      tunnel: w214 -> [w246 w265]
      tunnel: w209 -> [_ w260]
      frame False {
      }
      frame True {
        n96 = Get Date/Time In Seconds() -> (seconds since 1Jan1904=w278:timestamp)
        n97 = local read "Reset all"() -> (w262:bool)
        n98 = local read "Byte-Anzahl"() -> (w264:u32)
        n99 = local read "Start"() -> (w277:timestamp)
        n100 = VISA Read(VISA resource name=w283, byte count=w264, error in (no error)=w282) -> (VISA resource name out=w281:refnum<visa-resource-name>, read buffer=w280:string, error out=w273:errorcluster)  [unwired: 1 out]
        n101 = To Double Precision Float(number=w278) -> (double precision float=w274:dbl)
        n102 = Or(x=w262, y="Reset Spirometer") -> (x .or. y?=w261:bool)
        n103 = Scan Value(string=w280, format string="%.;%7.2" ("Format-String")) -> (value=w257:dbl)  [unwired: 1 in, 1 out]
        n104 = Or(x=w260, y=w261) -> (x .or. y?=w259:bool)
        n105 = To Double Precision Float(number=w277) -> (double precision float=w275:dbl)
        n106 = local read "Arraygröße"() -> (w258:i32)
        n107 = Subtract(x=w274, y=w275) -> (x-y=w251:dbl)
        "x-y 3" <- w251
        n108 = Add(x=w257, y=0.1336) -> (x+y=w255:dbl)
        n109 = Divide(x=w255, y=0.0218) -> (x/y=w252:dbl)
        "Vernier Spirometer" <- w252
        n110 = call "Build Vernier O4"("error in (no error)"=w273, "Reset"=w259, "Y Input"=w252, "X Input"=w274) -> ("error out"=w250:errorcluster, "XY Graph"=→"Vernier Spirometer":cluster{"X":dbl[], "Y":dbl[]}[])  [unwired: 6 in]
        n111 = Build Array(w251, w252) -> (w272:dbl[])
        "Current Value - \nVernier Spirometer" <- w272
        n112 = Build Array (concatenate)(w265, w272) -> (w271:dbl[][])
        "Data Storage vector - \nVernier Spirometer" <- w271
        n113 = Array Size(array=w271) -> (size(s)=w270:i32[])
        n114 = Index Array(array=w270, index=0 ("Index")) -> (element=w268:i32)
        "Vernier Spirometer-\n Array Größe" <- w268
        n115 = Greater Or Equal?(x=w268, y=w258) -> (x >= y?=w267:bool)
        n116 = case shown="True" w267 {
          tunnel: w271 -> [w284 w289]
          tunnel: [w284 w288] -> w266
          frame False {
          }
          frame True {
            n117 = Delete From Array(array=w289, length=1 ("Länge"), index (row)=0 ("Index")) -> (deleted portion=→"Gelöschte Elemente \nVernier Spirometer":dbl[][], array with subset deleted=w288:dbl[][])  [unwired: 1 in]
          }
        }
        n118 = call "Build Vernier O8"("error in (no error)"=w250, "Y Input"=w252, "X Input"=w251) -> ("error out"=w249:errorcluster, "XY Graph"=→"Vernier Spirometer - 2":cluster{"X":dbl[], "Y":dbl[]}[])  [unwired: 7 in]
      }
    }
    n119 = Select(t=dbl[][] [], s=w209, f=w211) -> (s? t:f=w208:dbl[][])
    n120 = feedback-in #2(w208) -> ()
    n121 = call <vilib>:"Simple Error Handler.vi"("type of dialog (OK msg:1)"=w216, "error in (no error)"=w219) -> ("error?"=w217:bool, "error out"=w215:errorcluster, "message"=→"Fehlermeldungen 6":string)  [unwired: 5 out]
    n122 = local read "Switch"() -> (w207:bool)
    n123 = case shown="False" w207 {
      frame False {
        n124 = for {
          N: 1 -> [_]
          n125 = property on="Vernier Spirometer - 2" class="XYGraph (strict)"("Visible"=FALSE) -> ()  [unwired: 2 in, 2 out]
          n126 = property on="Vernier Spirometer" class="XYGraph (strict)"("XScale.ScaleFit"=u8 2 ("X Scale.Scale Fit"), "XScale.FormatString"="%<%H:%M>T" ("X Scale.Format String"), "Visible"=TRUE) -> ()  [unwired: 2 in, 2 out]
        }
      }
      frame True {
        n127 = for {
          N: 1 -> [_]
          n128 = local read "x-y 3"() -> (w235:dbl)
          n129 = local read "Graph Range"() -> (w242:dbl)
          n130 = Subtract(x=w235, y=w242) -> (x-y=w241:dbl)
          n131 = Less Than 0?(x=w241) -> (x < 0?=w243:bool)
          n132 = case shown="False" w243 {
            tunnel: w241 -> [w244 _]
            tunnel: [w244 0.0] -> w240
            frame False {
            }
            frame True {
            }
          }
          n133 = property on="Vernier Spirometer" class="XYGraph (strict)"("Visible"=FALSE) -> ()  [unwired: 2 in, 2 out]
          n134 = property on="Vernier Spirometer - 2" class="XYGraph (strict)"("XScale.Maximum"=w235, "XScale.Minimum"=w240, "XScale.FormatString"="%u" ("X Scale.Format String"), "XScale.RngStart"=0.0 ("X Scale.Range:Start"), "Visible"=TRUE) -> ()  [unwired: 2 in, 2 out]
        }
      }
    }
  }
  n135 = while {
    tunnel: w28 -> [w310]
    tunnel: w27 -> [w309]
    tunnel: [w303] -> w26
    tunnel: [w298] -> w25
    stop <- w300 stop-if-true
    w299 = T1 0 items=["Kein Dialog", "OK-Meldung", "Dialog zum Fortsetzen oder Anhalten", "OK-Meldung + Warnungen", "Weiter/Stopp + Warnung"] ("type of dialog (OK msg:1)")
    w308 = u16 2 items=["None", "Last Bit", "TermChar"] ("Serial Settings:End Mode for Reads")
    n136 = Wait (ms)(milliseconds to wait=u32 200) -> ()  [unwired: 1 out]
    n137 = property class="Instr"(reference=w310, error in=w309, "TermChar En"=TRUE ("Message Based Settings:Termination Character Enable"), "ASRL End In"=w308) -> (reference out=w305:refnum<visa-resource-name>, error out=w304:errorcluster, "Serial Settings:Number of Bytes at Serial Port"=w307:u32)
    n138 = First Call?() -> (First Call?: T/F=w292:bool)
    n139 = Greater?(x=w307, y=u32 0) -> (0:w295:bool)
    n140 = feedback #3() -> (w297:dbl[][])  [unwired: 1 in]
    n141 = case shown="True" w295 {
      tunnel: w305 -> [w331 w362]
      tunnel: w304 -> [w330 w361]
      tunnel: [w331 w360] -> w303
      tunnel: [w330 w332] -> w302
      tunnel: [w329 w345] -> w294
      tunnel: w297 -> [w329 w344]
      tunnel: w292 -> [_ w339]
      frame False {
      }
      frame True {
        n142 = Get Date/Time In Seconds() -> (seconds since 1Jan1904=w357:timestamp)
        n143 = local read "Reset all"() -> (w341:bool)
        n144 = local read "Byte-Anzahl"() -> (w343:u32)
        n145 = local read "Start"() -> (w356:timestamp)
        n146 = VISA Read(VISA resource name=w362, byte count=w343, error in (no error)=w361) -> (VISA resource name out=w360:refnum<visa-resource-name>, read buffer=w359:string, error out=w352:errorcluster)  [unwired: 1 out]
        n147 = To Double Precision Float(number=w357) -> (double precision float=w353:dbl)
        n148 = Or(x=w341, y="Reset Vernier O2") -> (x .or. y?=w340:bool)
        n149 = Scan Value(string=w359, format string="%.;%7.2" ("Format-String")) -> (value=w334:dbl)  [unwired: 1 in, 1 out]
        "Vernier O2" <- w334
        n150 = Or(x=w339, y=w340) -> (x .or. y?=w338:bool)
        n151 = local read "Arraygröße"() -> (w337:i32)
        n152 = To Double Precision Float(number=w356) -> (double precision float=w354:dbl)
        n153 = call "Build Vernier O5"("error in (no error)"=w352, "Reset"=w338, "Y Input"=w334, "X Input"=w353) -> ("error out"=w333:errorcluster, "XY Graph"=→"Vernier O2":cluster{"X":dbl[], "Y":dbl[]}[])  [unwired: 6 in]
        n154 = Subtract(x=w353, y=w354) -> (x-y=w335:dbl)
        "x-y 2" <- w335
        n155 = Build Array(w335, w334) -> (w351:dbl[])
        "Current Value - Vernier O2" <- w351
        n156 = Build Array (concatenate)(w344, w351) -> (w350:dbl[][])
        "Vernier O2 - Data Storage Vector" <- w350
        n157 = Array Size(array=w350) -> (size(s)=w349:i32[])
        n158 = Index Array(array=w349, index=0 ("Index")) -> (element=w347:i32)
        "Vernier O2" <- w347
        n159 = Greater Or Equal?(x=w347, y=w337) -> (x >= y?=w346:bool)
        n160 = call "Build Vernier O7"("error in (no error)"=w333, "Y Input"=w334, "X Input"=w335) -> ("error out"=w332:errorcluster, "XY Graph"=→"Vernier O2 - 2":cluster{"X":dbl[], "Y":dbl[]}[])  [unwired: 7 in]
        n161 = case shown="False" w346 {
          tunnel: w350 -> [w363 w368]
          tunnel: [w363 w367] -> w345
          frame False {
          }
          frame True {
            n162 = Delete From Array(array=w368, length=1 ("Länge"), index (row)=0 ("Index")) -> (deleted portion=→"Gelöschte Elemente \nVernier O2":dbl[][], array with subset deleted=w367:dbl[][])  [unwired: 1 in]
          }
        }
      }
    }
    n163 = call <vilib>:"Simple Error Handler.vi"("type of dialog (OK msg:1)"=w299, "error in (no error)"=w302) -> ("error?"=w300:bool, "error out"=w298:errorcluster, "message"=→"Fehlermeldungen 7":string)  [unwired: 5 out]
    n164 = Select(t=dbl[][] [], s=w292, f=w294) -> (s? t:f=w293:dbl[][])
    n165 = feedback-in #3(w293) -> ()
    n166 = local read "Switch"() -> (w290:bool)
    n167 = case shown="False" w290 {
      frame False {
        n168 = for {
          N: 1 -> [_]
          n169 = property on="Vernier O2 - 2" class="XYGraph (strict)"("Visible"=FALSE) -> ()  [unwired: 2 in, 2 out]
          n170 = property on="Vernier O2" class="XYGraph (strict)"("XScale.ScaleFit"=u8 2 ("X Scale.Scale Fit"), "XScale.FormatString"="%<%H:%M>T" ("X Scale.Format String"), "Visible"=TRUE) -> ()  [unwired: 2 in, 2 out]
        }
      }
      frame True {
        n171 = for {
          N: 1 -> [_]
          n172 = local read "x-y 2"() -> (w318:dbl)
          n173 = local read "Graph Range"() -> (w326:dbl)
          n174 = Subtract(x=w318, y=w326) -> (x-y=w323:dbl)
          n175 = Less Than 0?(x=w323) -> (x < 0?=w325:bool)
          n176 = case shown="True" w325 {
            tunnel: w323 -> [w327 _]
            tunnel: [w327 0.0] -> w324
            frame False {
            }
            frame True {
            }
          }
          n177 = property on="Vernier O2" class="XYGraph (strict)"("Visible"=FALSE) -> ()  [unwired: 2 in, 2 out]
          n178 = property on="Vernier O2 - 2" class="XYGraph (strict)"("XScale.Maximum"=w318, "XScale.Minimum"=w324, "XScale.FormatString"="%u" ("X Scale.Format String"), "XScale.RngStart"=0.0 ("X Scale.Range:Start"), "Visible"=TRUE) -> ()  [unwired: 2 in, 2 out]
        }
      }
    }
  }
  n179 = while {
    tunnel: w42 -> [w389]
    tunnel: w41 -> [w388]
    tunnel: [w382] -> w44
    tunnel: [w377] -> w43
    stop <- w379 stop-if-true
    w378 = T1 0 items=["Kein Dialog", "OK-Meldung", "Dialog zum Fortsetzen oder Anhalten", "OK-Meldung + Warnungen", "Weiter/Stopp + Warnung"] ("type of dialog (OK msg:1)")
    w387 = u16 2 items=["None", "Last Bit", "TermChar"] ("Serial Settings:End Mode for Reads")
    n180 = Wait (ms)(milliseconds to wait=u32 200) -> ()  [unwired: 1 out]
    n181 = property class="Instr"(reference=w389, error in=w388, "TermChar En"=TRUE ("Message Based Settings:Termination Character Enable"), "ASRL End In"=w387) -> (reference out=w384:refnum<visa-resource-name>, error out=w383:errorcluster, "Serial Settings:Number of Bytes at Serial Port"=w386:u32)
    n182 = First Call?() -> (First Call?: T/F=w371:bool)
    n183 = Greater?(x=w386, y=u32 0) -> (0:w370:bool)
    n184 = feedback #4() -> (w376:dbl[][])  [unwired: 1 in]
    n185 = case shown="True" w370 {
      tunnel: w384 -> [w410 w441]
      tunnel: w383 -> [w409 w440]
      tunnel: [w410 w439] -> w382
      tunnel: [w409 w413] -> w381
      tunnel: [w408 w424] -> w374
      tunnel: w376 -> [w408 w423]
      tunnel: w371 -> [_ w418]
      frame False {
      }
      frame True {
        n186 = Get Date/Time In Seconds() -> (seconds since 1Jan1904=w436:timestamp)
        n187 = local read "Reset all"() -> (w420:bool)
        n188 = local read "Byte-Anzahl"() -> (w422:u32)
        n189 = local read "Start"() -> (w435:timestamp)
        n190 = VISA Read(VISA resource name=w441, byte count=w422, error in (no error)=w440) -> (VISA resource name out=w439:refnum<visa-resource-name>, read buffer=w438:string, error out=w431:errorcluster)  [unwired: 1 out]
        n191 = To Double Precision Float(number=w436) -> (double precision float=w432:dbl)
        n192 = Or(x=w420, y="Reset Vernier CO2") -> (x .or. y?=w419:bool)
        n193 = Scan Value(string=w438, format string="%.;%7.2" ("Format-String")) -> (value=w411:dbl)  [unwired: 1 in, 1 out]
        "Vernier CO2" <- w411
        n194 = Or(x=w418, y=w419) -> (x .or. y?=w417:bool)
        n195 = To Double Precision Float(number=w435) -> (double precision float=w433:dbl)
        n196 = local read "Arraygröße"() -> (w416:i32)
        n197 = call "Build Vernier O3"("error in (no error)"=w431, "Reset"=w417, "Y Input"=w411, "X Input"=w432) -> ("error out"=w414:errorcluster, "XY Graph"=→"Vernier CO2":cluster{"X":dbl[], "Y":dbl[]}[])  [unwired: 6 in]
        n198 = Subtract(x=w432, y=w433) -> (x-y=w412:dbl)
        "x-y 4" <- w412
        n199 = Build Array(w412, w411) -> (w430:dbl[])
        "Current Value Vernier CO2" <- w430
        n200 = Build Array (concatenate)(w423, w430) -> (w429:dbl[][])
        "Data Storage Vector - Vernier CO2" <- w429
        n201 = Array Size(array=w429) -> (size(s)=w428:i32[])
        n202 = Index Array(array=w428, index=0 ("Index")) -> (element=w426:i32)
        "Vernier CO2" <- w426
        n203 = Greater Or Equal?(x=w426, y=w416) -> (x >= y?=w425:bool)
        n204 = call "Build Vernier O9"("error in (no error)"=w414, "Y Input"=w411, "X Input"=w412) -> ("error out"=w413:errorcluster, "XY Graph"=→"Vernier CO2  - 2":cluster{"X":dbl[], "Y":dbl[]}[])  [unwired: 7 in]
        n205 = case shown="True" w425 {
          tunnel: w429 -> [w442 w447]
          tunnel: [w442 w446] -> w424
          frame False {
          }
          frame True {
            n206 = Delete From Array(array=w447, length=1 ("Länge"), index (row)=0 ("Index")) -> (deleted portion=→"Gelöschte Elemente \nVernier CO2":dbl[][], array with subset deleted=w446:dbl[][])  [unwired: 1 in]
          }
        }
      }
    }
    n207 = call <vilib>:"Simple Error Handler.vi"("type of dialog (OK msg:1)"=w378, "error in (no error)"=w381) -> ("error?"=w379:bool, "error out"=w377:errorcluster, "message"=→"Fehlermeldungen 4":string)  [unwired: 5 out]
    n208 = Select(t=dbl[][] [], s=w371, f=w374) -> (s? t:f=w372:dbl[][])
    n209 = feedback-in #4(w372) -> ()
    n210 = local read "Switch"() -> (w369:bool)
    n211 = case shown="False" w369 {
      frame False {
        n212 = for {
          N: 1 -> [_]
          n213 = property on="Vernier CO2  - 2" class="XYGraph (strict)"("Visible"=FALSE) -> ()  [unwired: 2 in, 2 out]
          n214 = property on="Vernier CO2" class="XYGraph (strict)"("XScale.ScaleFit"=u8 2 ("X Scale.Scale Fit"), "XScale.FormatString"="%<%H:%M>T" ("X Scale.Format String"), "Visible"=TRUE) -> ()  [unwired: 2 in, 2 out]
        }
      }
      frame True {
        n215 = for {
          N: 1 -> [_]
          n216 = local read "x-y 4"() -> (w402:dbl)
          n217 = local read "Graph Range"() -> (w403:dbl)
          n218 = Subtract(x=w402, y=w403) -> (x-y=w404:dbl)
          n219 = Less Than 0?(x=w404) -> (x < 0?=w405:bool)
          n220 = case shown="False" w405 {
            tunnel: w404 -> [w406 _]
            tunnel: [w406 0.0] -> w401
            frame False {
            }
            frame True {
            }
          }
          n221 = property on="Vernier CO2" class="XYGraph (strict)"("Visible"=FALSE) -> ()  [unwired: 2 in, 2 out]
          n222 = property on="Vernier CO2  - 2" class="XYGraph (strict)"("XScale.Maximum"=w402, "XScale.Minimum"=w401, "XScale.FormatString"="%u" ("X Scale.Format String"), "XScale.RngStart"=0.0 ("X Scale.Range:Start"), "Visible"=TRUE) -> ()  [unwired: 2 in, 2 out]
        }
      }
    }
  }
  n223 = while {
    tunnel: w36 -> [w468]
    tunnel: w35 -> [w467]
    tunnel: [w461] -> w34
    tunnel: [w456] -> w33
    stop <- w458 stop-if-true
    w457 = T1 0 items=["Kein Dialog", "OK-Meldung", "Dialog zum Fortsetzen oder Anhalten", "OK-Meldung + Warnungen", "Weiter/Stopp + Warnung"] ("type of dialog (OK msg:1)")
    w466 = u16 2 items=["None", "Last Bit", "TermChar"] ("Serial Settings:End Mode for Reads")
    n224 = Wait (ms)(milliseconds to wait=u32 200) -> ()  [unwired: 1 out]
    n225 = property class="Instr"(reference=w468, error in=w467, "TermChar En"=TRUE ("Message Based Settings:Termination Character Enable"), "ASRL End In"=w466) -> (reference out=w463:refnum<visa-resource-name>, error out=w462:errorcluster, "Serial Settings:Number of Bytes at Serial Port"=w465:u32)
    n226 = First Call?() -> (First Call?: T/F=w450:bool)
    n227 = Greater?(x=w465, y=u32 0) -> (0:w449:bool)
    n228 = feedback #5() -> (w455:dbl[][])  [unwired: 1 in]
    n229 = case shown="True" w449 {
      tunnel: w463 -> [w489 w520]
      tunnel: w462 -> [w488 w519]
      tunnel: [w489 w518] -> w461
      tunnel: [w488 w492] -> w460
      tunnel: [w487 w503] -> w453
      tunnel: w455 -> [w487 w502]
      tunnel: w450 -> [_ w497]
      frame False {
      }
      frame True {
        n230 = Get Date/Time In Seconds() -> (seconds since 1Jan1904=w515:timestamp)
        n231 = local read "Reset all"() -> (w499:bool)
        n232 = local read "Byte-Anzahl"() -> (w501:u32)
        n233 = local read "Start"() -> (w514:timestamp)
        n234 = VISA Read(VISA resource name=w520, byte count=w501, error in (no error)=w519) -> (VISA resource name out=w518:refnum<visa-resource-name>, read buffer=w517:string, error out=w510:errorcluster)  [unwired: 1 out]
        n235 = To Double Precision Float(number=w515) -> (double precision float=w511:dbl)
        n236 = Or(x=w499, y="Reset MHZ19b") -> (x .or. y?=w498:bool)
        n237 = Scan Value(string=w517, format string="%.;%7.2" ("Format-String")) -> (value=w490:dbl)  [unwired: 1 in, 1 out]
        "MHZ19b" <- w490
        n238 = Or(x=w497, y=w498) -> (x .or. y?=w496:bool)
        n239 = To Double Precision Float(number=w514) -> (double precision float=w512:dbl)
        n240 = local read "Arraygröße"() -> (w495:i32)
        n241 = call "Build Vernier O"("error in (no error)"=w510, "Reset"=w496, "Y Input"=w490, "X Input"=w511) -> ("error out"=w493:errorcluster, "XY Graph"=→"MH-Z19B":cluster{"X":dbl[], "Y":dbl[]}[])  [unwired: 6 in]
        n242 = Subtract(x=w511, y=w512) -> (x-y=w491:dbl)
        "x-y 5" <- w491
        n243 = Build Array(w491, w490) -> (w509:dbl[])
        "Current Value - MHZ19b" <- w509
        n244 = Build Array (concatenate)(w502, w509) -> (w508:dbl[][])
        "MHZ19b" <- w508
        n245 = Array Size(array=w508) -> (size(s)=w507:i32[])
        n246 = call "Build Vernier O10"("error in (no error)"=w493, "Y Input"=w490, "X Input"=w491) -> ("error out"=w492:errorcluster, "XY Graph"=→"MH-Z19B - 2":cluster{"X":dbl[], "Y":dbl[]}[])  [unwired: 7 in]
        n247 = Index Array(array=w507, index=0 ("Index")) -> (element=w505:i32)
        "MHZ19b - Arraygröße" <- w505
        n248 = Greater Or Equal?(x=w505, y=w495) -> (x >= y?=w504:bool)
        n249 = case shown="True" w504 {
          tunnel: w508 -> [w521 w526]
          tunnel: [w521 w525] -> w503
          frame False {
          }
          frame True {
            n250 = Delete From Array(array=w526, length=1 ("Länge"), index (row)=0 ("Index")) -> (deleted portion=→"Gelöschte Elemente \nMHZ19b":dbl[][], array with subset deleted=w525:dbl[][])  [unwired: 1 in]
          }
        }
      }
    }
    n251 = call <vilib>:"Simple Error Handler.vi"("type of dialog (OK msg:1)"=w457, "error in (no error)"=w460) -> ("error?"=w458:bool, "error out"=w456:errorcluster, "message"=→"Fehlermeldungen 5":string)  [unwired: 5 out]
    n252 = Select(t=dbl[][] [], s=w450, f=w453) -> (s? t:f=w451:dbl[][])
    n253 = feedback-in #5(w451) -> ()
    n254 = local read "Switch"() -> (w448:bool)
    n255 = case shown="True" w448 {
      frame False {
        n256 = for {
          N: 1 -> [_]
          n257 = property on="MH-Z19B - 2" class="XYGraph (strict)"("Visible"=FALSE) -> ()  [unwired: 2 in, 2 out]
          n258 = property on="MH-Z19B" class="XYGraph (strict)"("XScale.ScaleFit"=u8 2 ("X Scale.Scale Fit"), "XScale.FormatString"="%<%H:%M>T" ("X Scale.Format String"), "Visible"=TRUE) -> ()  [unwired: 2 in, 2 out]
        }
      }
      frame True {
        n259 = for {
          N: 1 -> [_]
          n260 = local read "x-y 5"() -> (w476:dbl)
          n261 = local read "Graph Range"() -> (w484:dbl)
          n262 = Subtract(x=w476, y=w484) -> (x-y=w482:dbl)
          n263 = Less Than 0?(x=w482) -> (x < 0?=w483:bool)
          n264 = property on="MH-Z19B" class="XYGraph (strict)"("Visible"=FALSE) -> ()  [unwired: 2 in, 2 out]
          n265 = case shown="False" w483 {
            tunnel: [w485 0.0] -> w477
            tunnel: w482 -> [w485 _]
            frame False {
            }
            frame True {
            }
          }
          n266 = property on="MH-Z19B - 2" class="XYGraph (strict)"("XScale.Maximum"=w476, "XScale.Minimum"=w477, "XScale.FormatString"="%u" ("X Scale.Format String"), "XScale.RngStart"=0.0 ("X Scale.Range:Start"), "Visible"=TRUE) -> ()  [unwired: 2 in, 2 out]
        }
      }
    }
  }
  n267 = while {
    tunnel: w4 -> [w543]
    tunnel: w3 -> [w542]
    tunnel: [w530] -> w8
    tunnel: [w528] -> w9
    stop <- w529 stop-if-true
    w532 = T1 0 items=["Kein Dialog", "OK-Meldung", "Dialog zum Fortsetzen oder Anhalten", "OK-Meldung + Warnungen", "Weiter/Stopp + Warnung"] ("type of dialog (OK msg:1)")
    w546 = u16 2 items=["None", "Last Bit", "TermChar"] ("Serial Settings:End Mode for Reads")
    n268 = Wait (ms)(milliseconds to wait=u32 200) -> ()  [unwired: 1 out]
    n269 = property class="Instr"(reference=w543, error in=w542, "TermChar En"=TRUE ("Message Based Settings:Termination Character Enable"), "ASRL End In"=w546) -> (reference out=w540:refnum<visa-resource-name>, error out=w539:errorcluster, "Serial Settings:Number of Bytes at Serial Port"=w545:u32)
    n270 = Greater?(x=w545, y=u32 0) -> (0:w541:bool)
    n271 = local read "Switch"() -> (w527:bool)
    n272 = case shown="False" w527 {
      frame False {
        n273 = for {
          N: 1 -> [_]
          w550 = FALSE
          w552 = u8 2 ("X Scale.Scale Fit")
          w553 = "%<%H:%M>T" ("X Scale.Format String")
          w551 = TRUE ("Visible")
          n274 = property on="eCO2" class="XYGraph (strict)"("Visible"=w551, "XScale.ScaleFit"=w552, "XScale.FormatString"=w553) -> ()  [unwired: 2 in, 2 out]
          n275 = property on="eCO2 - 2" class="XYGraph (strict)"("Visible"=w550) -> ()  [unwired: 2 in, 2 out]
          n276 = property on="TVOC" class="XYGraph (strict)"("Visible"=w551, "XScale.ScaleFit"=w552, "XScale.FormatString"=w553) -> ()  [unwired: 2 in, 2 out]
          n277 = property on="TVOC - 2" class="XYGraph (strict)"("Visible"=w550) -> ()  [unwired: 2 in, 2 out]
          n278 = property on="RAW H2" class="XYGraph (strict)"("Visible"=w551, "XScale.ScaleFit"=w552, "XScale.FormatString"=w553) -> ()  [unwired: 2 in, 2 out]
          n279 = property on="RAW H2 - 2" class="XYGraph (strict)"("Visible"=w550) -> ()  [unwired: 2 in, 2 out]
          n280 = property on="RAW Ethanol" class="XYGraph (strict)"("Visible"=w551, "XScale.ScaleFit"=w552, "XScale.FormatString"=w553) -> ()  [unwired: 2 in, 2 out]
          n281 = property on="RAW Ethanol - 2" class="XYGraph (strict)"("Visible"=w550) -> ()  [unwired: 2 in, 2 out]
          n282 = property on="Luftfeuchtigkeit" class="XYGraph (strict)"("Visible"=w551, "XScale.ScaleFit"=w552, "XScale.FormatString"=w553) -> ()  [unwired: 2 in, 2 out]
          n283 = property on="Luftfeuchtigkeit - 2" class="XYGraph (strict)"("Visible"=w550) -> ()  [unwired: 2 in, 2 out]
          n284 = property on="Temperatur" class="XYGraph (strict)"("Visible"=w551, "XScale.ScaleFit"=w552, "XScale.FormatString"=w553) -> ()  [unwired: 2 in, 2 out]
          n285 = property on="Temperatur - 2" class="XYGraph (strict)"("Visible"=w550) -> ()  [unwired: 2 in, 2 out]
          n286 = property on="MQ3" class="XYGraph (strict)"("Visible"=w551, "XScale.ScaleFit"=w552, "XScale.FormatString"=w553) -> ()  [unwired: 2 in, 2 out]
          n287 = property on="MQ3 - 2" class="XYGraph (strict)"("Visible"=w550) -> ()  [unwired: 2 in, 2 out]
          n288 = property on="MQ4" class="XYGraph (strict)"("Visible"=w551, "XScale.ScaleFit"=w552, "XScale.FormatString"=w553) -> ()  [unwired: 2 in, 2 out]
          n289 = property on="MQ4 - 2" class="XYGraph (strict)"("Visible"=w550) -> ()  [unwired: 2 in, 2 out]
        }
      }
      frame True {
        n290 = for {
          N: 1 -> [_]
          w555 = TRUE
          w556 = FALSE
          w557 = "%u"
          w558 = 0.0
          n291 = local read "Graph Range"() -> (w562:dbl)
          n292 = local read "x-y 6"() -> (w559:dbl)
          n293 = Subtract(x=w559, y=w562) -> (x-y=w561:dbl)
          n294 = Less Than 0?(x=w561) -> (x < 0?=w563:bool)
          n295 = case shown="True" w563 {
            tunnel: w561 -> [w564 _]
            tunnel: [w564 0.0] -> w560
            frame False {
            }
            frame True {
            }
          }
          n296 = property on="eCO2 - 2" class="XYGraph (strict)"("XScale.Maximum"=w559, "XScale.Minimum"=w560, "XScale.FormatString"=w557, "XScale.RngStart"=w558, "Visible"=w555) -> ()  [unwired: 2 in, 2 out]
          n297 = property on="eCO2" class="XYGraph (strict)"("Visible"=w556) -> ()  [unwired: 2 in, 2 out]
          n298 = property on="TVOC" class="XYGraph (strict)"("Visible"=w556) -> ()  [unwired: 2 in, 2 out]
          n299 = property on="TVOC - 2" class="XYGraph (strict)"("XScale.Maximum"=w559, "XScale.Minimum"=w560, "XScale.FormatString"=w557, "XScale.RngStart"=w558, "Visible"=w555) -> ()  [unwired: 2 in, 2 out]
          n300 = property on="RAW H2" class="XYGraph (strict)"("Visible"=w556) -> ()  [unwired: 2 in, 2 out]
          n301 = property on="RAW H2 - 2" class="XYGraph (strict)"("XScale.Maximum"=w559, "XScale.Minimum"=w560, "XScale.FormatString"=w557, "XScale.RngStart"=w558, "Visible"=w555) -> ()  [unwired: 2 in, 2 out]
          n302 = property on="RAW Ethanol" class="XYGraph (strict)"("Visible"=w556) -> ()  [unwired: 2 in, 2 out]
          n303 = property on="RAW Ethanol - 2" class="XYGraph (strict)"("XScale.Maximum"=w559, "XScale.Minimum"=w560, "XScale.FormatString"=w557, "XScale.RngStart"=w558, "Visible"=w555) -> ()  [unwired: 2 in, 2 out]
          n304 = property on="Luftfeuchtigkeit" class="XYGraph (strict)"("Visible"=w556) -> ()  [unwired: 2 in, 2 out]
          n305 = property on="Luftfeuchtigkeit - 2" class="XYGraph (strict)"("XScale.Maximum"=w559, "XScale.Minimum"=w560, "XScale.FormatString"=w557, "XScale.RngStart"=w558, "Visible"=w555) -> ()  [unwired: 2 in, 2 out]
          n306 = property on="Temperatur - 2" class="XYGraph (strict)"("XScale.Maximum"=w559, "XScale.Minimum"=w560, "XScale.FormatString"=w557, "XScale.RngStart"=w558, "Visible"=w555) -> ()  [unwired: 2 in, 2 out]
          n307 = property on="Temperatur" class="XYGraph (strict)"("Visible"=w556) -> ()  [unwired: 2 in, 2 out]
          n308 = property on="MQ3 - 2" class="XYGraph (strict)"("XScale.Maximum"=w559, "XScale.Minimum"=w560, "XScale.FormatString"=w557, "XScale.RngStart"=w558, "Visible"=w555) -> ()  [unwired: 2 in, 2 out]
          n309 = property on="MQ3" class="XYGraph (strict)"("Visible"=w556) -> ()  [unwired: 2 in, 2 out]
          n310 = property on="MQ4 - 2" class="XYGraph (strict)"("XScale.Maximum"=w559, "XScale.Minimum"=w560, "XScale.FormatString"=w557, "XScale.RngStart"=w558, "Visible"=w555) -> ()  [unwired: 2 in, 2 out]
          n311 = property on="MQ4" class="XYGraph (strict)"("Visible"=w556) -> ()  [unwired: 2 in, 2 out]
        }
      }
    }
    n312 = feedback #6() -> (w538:dbl[][])  [unwired: 1 in]
    n313 = case shown="True" w541 {
      tunnel: w540 -> [w567 w683]
      tunnel: w539 -> [w566 w682]
      tunnel: [w568 w634] -> w537
      tunnel: w538 -> [w568 w639]
      tunnel: [w566 w633] -> w531
      tunnel: [w567 w632] -> w528
      frame False {
      }
      frame True {
        n314 = local read "Reset all"() -> (w630:bool)
        n315 = local read "Reset all"() -> (w628:bool)
        n316 = local read "Reset all"() -> (w625:bool)
        n317 = local read "Reset all"() -> (w624:bool)
        n318 = local read "Reset all"() -> (w622:bool)
        n319 = local read "Reset all"() -> (w604:bool)
        n320 = local read "Reset all"() -> (w606:bool)
        n321 = local read "Start"() -> (w643:timestamp)
        n322 = local read "Byte-Anzahl"() -> (w681:u32)
        n323 = VISA Read(VISA resource name=w683, byte count=w681, error in (no error)=w682) -> (VISA resource name out=w632:refnum<visa-resource-name>, read buffer=w674:string, error out=w633:errorcluster)  [unwired: 1 out]
        n324 = Or(x=w630, y="reset eCO2") -> (x .or. y?=w619:bool)
        n325 = Or(x=w628, y="reset TVOC") -> (x .or. y?=w617:bool)
        n326 = Or(x=w625, y="Reset RAW H2") -> (x .or. y?=w615:bool)
        n327 = Or(x=w624, y="Reset RAW Ethanol") -> (x .or. y?=w613:bool)
        n328 = Or(x=w622, y="Reset Luftfeuchtigkeit") -> (x .or. y?=w611:bool)
        n329 = Or(x=w606, y="Reset MQ4") -> (x .or. y?=w607:bool)
        n330 = First Call?() -> (First Call?: T/F=w610:bool)
        n331 = Get Date/Time In Seconds() -> (seconds since 1Jan1904=w642:timestamp)
        n332 = First Call?() -> (First Call?: T/F=w620:bool)
        n333 = Or(x=w604, y="Reset MQ3") -> (x .or. y?=w609:bool)
        n334 = First Call?() -> (First Call?: T/F=w608:bool)
        n335 = First Call?() -> (First Call?: T/F=w616:bool)
        n336 = First Call?() -> (First Call?: T/F=w618:bool)
        n337 = First Call?() -> (First Call?: T/F=w614:bool)
        n338 = First Call?() -> (First Call?: T/F=w612:bool)
        n339 = Or(x=w620, y=w619) -> (x .or. y?=w602:bool)
        n340 = Or(x=w618, y=w617) -> (x .or. y?=w601:bool)
        n341 = Or(x=w616, y=w615) -> (x .or. y?=w600:bool)
        n342 = Or(x=w614, y=w613) -> (x .or. y?=w599:bool)
        n343 = Or(x=w612, y=w611) -> (x .or. y?=w598:bool)
        n344 = Or(x=w610, y=w609) -> (x .or. y?=w597:bool)
        n345 = Or(x=w608, y=w607) -> (x .or. y?=w596:bool)
        n346 = To Double Precision Float(number=w642) -> (double precision float=w591:dbl)
        n347 = To Double Precision Float(number=w643) -> (double precision float=w641:dbl)
        n348 = Subtract(x=w591, y=w641) -> (x-y=w579:dbl)
        "x-y 6" <- w579
        n349 = Match Pattern(string=w674, regular expression="", offset (0)=4) -> (after substring=w676:string)  [unwired: 3 out]
        n350 = Match Pattern(string=w676, regular expression="TVOC:") -> (before substring=w678:string, after substring=w673:string)  [unwired: 1 in, 2 out]
        n351 = Match Pattern(string=w673, regular expression="Raw H2:") -> (before substring=w671:string, after substring=w667:string)  [unwired: 1 in, 2 out]
        n352 = Scan Value(string=w678, format string="%4") -> (value=w584:dbl)  [unwired: 1 in, 1 out]
        "eCO2" <- w584
        n353 = Match Pattern(string=w667, regular expression="Raw Ethanol:") -> (before substring=w665:string, after substring=w662:string)  [unwired: 1 in, 2 out]
        n354 = call "Build eCO"("Reset"=w602, "Y Input"=w584, "X Input"=w591) -> ("XY Graph"=→"eCO2":cluster{"X":dbl[], "Y":dbl[]}[])  [unwired: 7 in, 1 out]
        n355 = Scan Value(string=w671, format string="%4") -> (value=w582:dbl)  [unwired: 1 in, 1 out]
        "TVOC" <- w582
        n356 = Match Pattern(string=w662, regular expression="Luftfeuchtigkeit:") -> (before substring=w659:string, after substring=w631:string)  [unwired: 1 in, 2 out]
        n357 = Scan Value(string=w665, format string="%5") -> (value=w587:dbl)  [unwired: 1 in, 1 out]
        n358 = Scan Value(string=w659, format string="%5") -> (value=w589:dbl)  [unwired: 1 in, 1 out]
        n359 = Divide(x=w587, y=1000.0) -> (x/y=w580:dbl)
        "RAW H2" <- w580
        n360 = call "Build TVOC"("Reset"=w601, "Y Input"=w582, "X Input"=w591) -> ("XY Graph"=→"TVOC":cluster{"X":dbl[], "Y":dbl[]}[])  [unwired: 7 in, 1 out]
        n361 = Match Pattern(string=w631, regular expression="Temperatur:") -> (before substring=w655:string, after substring=w653:string)  [unwired: 1 in, 2 out]
        n362 = Divide(x=w589, y=1000.0) -> (x/y=w573:dbl)
        "RAW Ethanol" <- w573
        n363 = call "RAW H"("Reset"=w600, "Y Input"=w580, "X Input"=w591) -> ("XY Graph"=→"RAW H2":cluster{"X":dbl[], "Y":dbl[]}[])  [unwired: 7 in, 1 out]
        n364 = call "Build RAW Ethanol"("Reset"=w599, "Y Input"=w573, "X Input"=w591) -> ("XY Graph"=→"RAW Ethanol":cluster{"X":dbl[], "Y":dbl[]}[])  [unwired: 7 in, 1 out]
        n365 = Match Pattern(string=w653, regular expression="MQ3:") -> (before substring=w593:string, after substring=w650:string)  [unwired: 1 in, 2 out]
        n366 = Scan Value(string=w655, format string="%.;%4.2f") -> (value=w572:dbl)  [unwired: 1 in, 1 out]
        "Luftfeuchtigkeit" <- w572
        n367 = Scan Value(string=w593, format string="%.;%4.2f") -> (value=w571:dbl)  [unwired: 1 in, 1 out]
        "Temperatur" <- w571
        n368 = Match Pattern(string=w650, regular expression="MQ4:") -> (before substring=w649:string, after substring=w648:string)  [unwired: 1 in, 2 out]
        n369 = call "Build Luftfeuchtigkeit2"("Y Input"=w571, "X Input"=w591) -> ("XY Graph"=→"Temperatur":cluster{"X":dbl[], "Y":dbl[]}[])  [unwired: 8 in, 1 out]
        n370 = call "Build Luftfeuchtigkeit"("Reset"=w598, "Y Input"=w572, "X Input"=w591) -> ("XY Graph"=→"Luftfeuchtigkeit":cluster{"X":dbl[], "Y":dbl[]}[])  [unwired: 7 in, 1 out]
        n371 = Scan Value(string=w648, format string="%4") -> (value=w569:dbl)  [unwired: 1 in, 1 out]
        "MQ4" <- w569
        n372 = Scan Value(string=w649, format string="%4") -> (value=w570:dbl)  [unwired: 1 in, 1 out]
        "MQ3" <- w570
        n373 = call "Build MQ3"("Reset"=w597, "Y Input"=w570, "X Input"=w591) -> ("XY Graph"=→"MQ3":cluster{"X":dbl[], "Y":dbl[]}[])  [unwired: 7 in, 1 out]
        n374 = call "Build MQ4"("Reset"=w596, "Y Input"=w569, "X Input"=w591) -> ("XY Graph"=→"MQ4":cluster{"X":dbl[], "Y":dbl[]}[])  [unwired: 7 in, 1 out]
        n375 = Build Array(w579, w584, w582, w580, w573, w572, w570, w569) -> (w640:dbl[])
        "Current Value HEMTLL" <- w640
        n376 = call "Build TVOC2"("Y Input"=w582, "X Input"=w579) -> ("XY Graph"=→"TVOC - 2":cluster{"X":dbl[], "Y":dbl[]}[])  [unwired: 8 in, 1 out]
        n377 = call "RAW H2"("Y Input"=w580, "X Input"=w579) -> ("XY Graph"=→"RAW H2 - 2":cluster{"X":dbl[], "Y":dbl[]}[])  [unwired: 8 in, 1 out]
        n378 = call "Build RAW Ethanol2"("Y Input"=w573, "X Input"=w579) -> ("XY Graph"=→"RAW Ethanol - 2":cluster{"X":dbl[], "Y":dbl[]}[])  [unwired: 8 in, 1 out]
        n379 = call "Build RAW Ethanol3"("Y Input"=w572, "X Input"=w579) -> ("XY Graph"=→"Luftfeuchtigkeit - 2":cluster{"X":dbl[], "Y":dbl[]}[])  [unwired: 8 in, 1 out]
        n380 = call "Build RAW Ethanol4"("Y Input"=w571, "X Input"=w579) -> ("XY Graph"=→"Temperatur - 2":cluster{"X":dbl[], "Y":dbl[]}[])  [unwired: 8 in, 1 out]
        n381 = call "Build RAW Ethanol5"("Y Input"=w570, "X Input"=w579) -> ("XY Graph"=→"MQ3 - 2":cluster{"X":dbl[], "Y":dbl[]}[])  [unwired: 8 in, 1 out]
        n382 = call "Build RAW Ethanol6"("Y Input"=w569, "X Input"=w579) -> ("XY Graph"=→"MQ4 - 2":cluster{"X":dbl[], "Y":dbl[]}[])  [unwired: 8 in, 1 out]
        n383 = call "Build eCO2"("Y Input"=w584, "X Input"=w579) -> ("XY Graph"=→"eCO2 - 2":cluster{"X":dbl[], "Y":dbl[]}[])  [unwired: 8 in, 1 out]
        n384 = Build Array (concatenate)(w639, w640) -> (w635:dbl[][])
        "Data Storage Vector - HEMTLL" <- w635
        n385 = Array Size(array=w635) -> (size(s)=w638:i32[])
        n386 = local read "Arraygröße"() -> (w594:i32)
        n387 = Index Array(array=w638, index=0 ("Index")) -> (element=w595:i32)
        "HEMTLL - Arraygröße" <- w595
        n388 = Greater Or Equal?(x=w595, y=w594) -> (x >= y?=w636:bool)
        n389 = case shown="True" w636 {
          tunnel: w635 -> [w684 w687]
          tunnel: [w684 w686] -> w634
          frame False {
          }
          frame True {
            n390 = Delete From Array(array=w687, length=1 ("Länge"), index (row)=0 ("Index")) -> (deleted portion=→"Gelöschte Elemente\nHEMTTL":dbl[][], array with subset deleted=w686:dbl[][])  [unwired: 1 in]
          }
        }
      }
    }
    n391 = First Call?() -> (First Call?: T/F=w534:bool)
    n392 = call <vilib>:"Simple Error Handler.vi"("type of dialog (OK msg:1)"=w532, "error in (no error)"=w531) -> ("error?"=w529:bool, "error out"=w530:errorcluster, "message"=→"Fehlermeldungen 8":string)  [unwired: 5 out]
    n393 = Select(t=dbl[][] [], s=w534, f=w537) -> (s? t:f=w535:dbl[][])
    n394 = feedback-in #6(w535) -> ()
  }
  n395 = VISA Close(VISA resource name=w32, error in (no error)=w31) -> (error out=w2:errorcluster)
  n396 = VISA Close(VISA resource name=w34, error in (no error)=w33) -> ()  [unwired: 1 out]
  n397 = VISA Close(VISA resource name=w44, error in (no error)=w43) -> ()  [unwired: 1 out]
  n398 = VISA Close(VISA resource name=w26, error in (no error)=w25) -> ()  [unwired: 1 out]
  n399 = call <vilib>:"Simple Error Handler.vi"("type of dialog (OK msg:1)"=w1, "error in (no error)"=w2) -> ()  [unwired: 8 out]
  n400 = VISA Close(VISA resource name=w79, error in (no error)=w78) -> ()  [unwired: 1 out]
  n401 = VISA Close(VISA resource name=w9, error in (no error)=w8) -> ()  [unwired: 1 out]
